vi "DMM.vi"(11 "Queue Ref In":T1={"UI"=refnum, "Message"=refnum, "Data"=refnum, "Caller"=refnum, "Name"="000 Common", "Data Path"=path "", "Class Path"=path "", "SubPanel"=refnum, "Project Name"="", "MNT"="", "Title"="", "Data Source"=refnum, "Queue List"={}, "VI"=refnum, "UE"=refnum}) -> ()   [LabVIEW 2020]
doc: "Digital Multimeter"
uses:
  <vilib>/Retry/UI Control Suite/Boolean/System Buttons/Connect Button.ctl
  <vilib>/Retry/UI Control Suite/Boolean/System Buttons/Acquire Button.ctl
  <vilib>/Retry/UI Control Suite/Boolean/System Buttons/Upload Button.ctl
  <vilib>/Retry/UI Control Suite/Boolean/System Buttons/Update Button.ctl
  <vilib>/Retry/UI Control Suite/Boolean/System Buttons/Excel Button.ctl
  <vilib>/Retry/MListBox/MListBox.lvclass
  <vilib>/Retry/MListBox/Type Definitions/Autosize Mode.ctl
  <vilib>/Retry/MListBox/MListBox.lvclass/MListBox.ctl
  <userlib>/_OpenG.lib/array/array.llb/Filter 1D Array with Scalar (I32)__ogtk.vi
  <userlib>/_OpenG.lib/array/array.llb/Sort 2D Array (String)__ogtk.vi
  Spire.XLS.dll
  <vilib>/Retry/Spire Excel/Spire_Excel.lvlib
  <instrlib>/Fluke 5XXX Series Multicalibrators/Fluke 5XXX Series Multicalibrators.lvlib
panel:
  in  "待选参数":i32[](listbox)
  in  "Title":string="数字多用表自动化计量软件V1.0"
  in  "打开报告":T2
  in  "复位":T3
  in  "暂停":bool
  in  "测量参数":T4={"电阻"=TRUE, "直流电压"=TRUE, "交流电压"=TRUE, "直流电流"=TRUE, "交流电流"=TRUE}
  in  "样品编号":string
  in  "载入模版":T5
  in  "型号":u16(ring) items=["34401A", "34461A", "Simulation DMM"]
  in  "保存":bool
  in  "测量":T6
  out "Connected?":bool
  in  "连接":T7
  in  "源地址":refnum<visa-resource-name>="GPIB0::4::INSTR"
  in  "数表地址":refnum<visa-resource-name>
  in  "Tab Control":enum32{"直流电压", "直流电流", "交流电压", "交流电流", "电阻"}(tab)
  in  "直流电压_MLb":i32(listbox)
  in  "直流电流_MLb":i32(listbox)
  in  "交流电压_MLb":i32(listbox)
  in  "交流电流_MLb":i32(listbox)
  in  "电阻_MLb":i32(listbox)
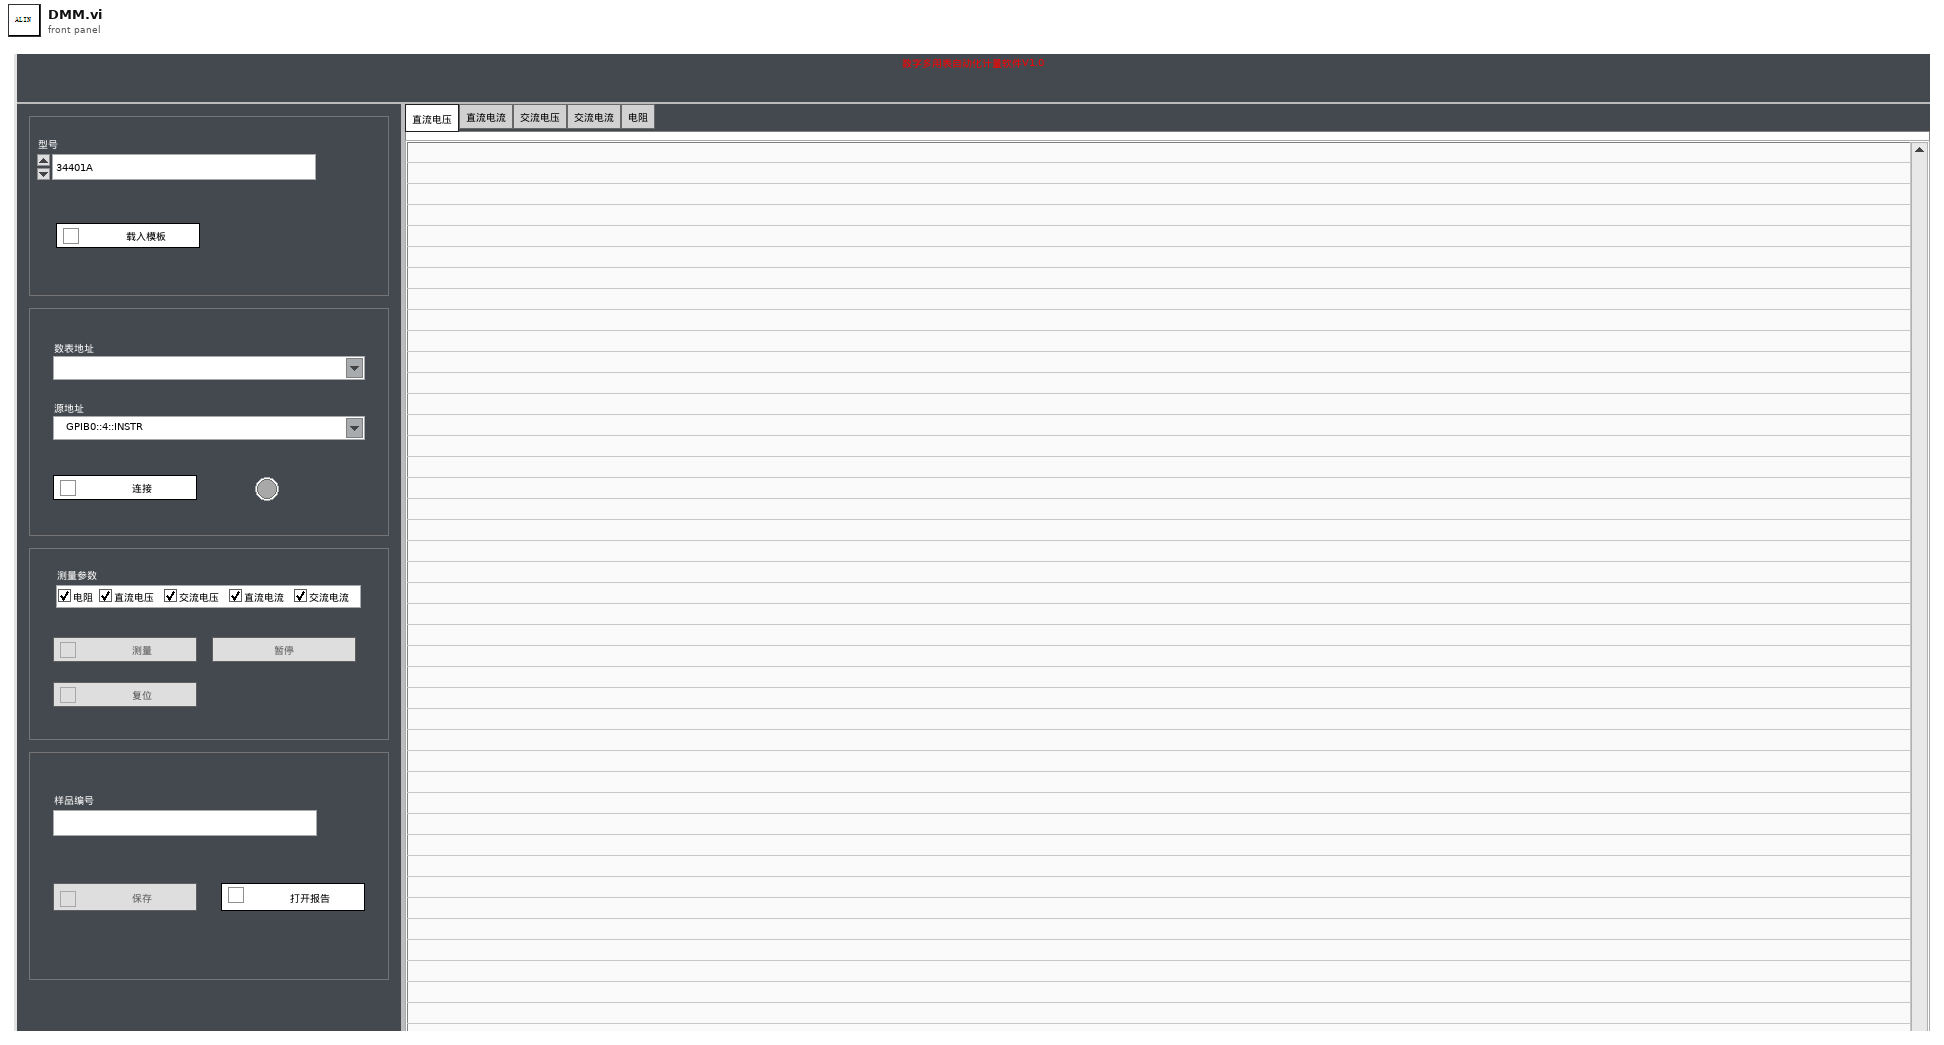
[diagram p1: front panel]
types:
  T1 = typedef "000 Module Data Type.ctl" = cluster{"UI":refnum<queue>, "Message":refnum<queue>, "Data":refnum<queue>, "Caller":refnum<queue>, "Name":string, "Data Path":path, "Class Path":path, "SubPanel":refnum<vi>, "Project Name":string, "MNT":string, "Title":string, "Data Source":refnum<queue>, "Queue List":map{string, refnum<queue>}, "VI":refnum<vi>, "UE":refnum<user-event>}
  T2 = typedef "Excel Button.ctl" = bool
  T3 = typedef "Update Button.ctl" = bool
  T4 = cluster{"电阻":bool, "直流电压":bool, "交流电压":bool, "直流电流":bool, "交流电流":bool}
  T5 = typedef "Upload Button.ctl" = bool
  T6 = typedef "Acquire Button.ctl" = bool
  T7 = typedef "Connect Button.ctl" = bool
  T8 = cluster{"Queue":T1, "Delay":cluster{"Count Time(ms)":u32, "Delay Time(ms)":u32, "Next":string}, "connection ID":refnum<k5>, "Save path":path, "testCount":u32, "数字多用表接口":refnum<class "数字多用表接口.lvclass">, "多功能校准源接口":refnum<class "多功能校准源接口.lvclass">, "workbook":refnum<k24>, "点数范围":string[][], "参数个数":string[], "当前参数":string, "个数索引":i32, "配置数组":string[][], "Measurement":dbl, "MLbs":refnum<class "MListBox.lvclass">[], "测量参数":refnum<vi>, "测量参数s":string[], "参数索引":i32, "接线状态":cluster{"上次接线状态":i32, "当前接线状态":i32}, "MListBox":refnum<class "MListBox.lvclass">, "初始化数据":string[][][], "Message":string, "Delay Time(ms)":u32, "MeaCount":i32, "Restart":bool}
  T9 = enum8{"Enabled", "Disabled", "Disabled and Grayed Out"}
  T10 = enum16{"DC Voltage", "AC Voltage", "Resistance", "DC Current", "AC Current"}
  T11 = typedef "Autosize Mode.ctl" = enum16{"Header", "All Cells"}
  T12 = cluster{"MListBox":refnum<class "MListBox.lvclass">, "Values":string[][]}
  T13 = cluster{"Queue":T1, "MLbs":refnum<class "MListBox.lvclass">[], "MListBox":refnum<class "MListBox.lvclass">}
  T14 = enum32{"invalid app kind", "Development System", "Run Time System", "Student Edition", "Embedded LabVIEW", "Evaluation", "Custom"}
  T15 = typedef "eventvkey.ctl" = enum16{"ASCII", "Enter", "Return", "Shift", "Ctrl", "Alt", "Cmd", "Opt", "Caps", "NumLock", "Clear", "Break", "Up", "Down", "Left", "Right", "Insert", "Delete", "Home", "End", "PageUp", "PageDown", "Escape", "Help", "Pause", "ScrollLock", "F1", "F2", "F3", "F4", "F5", "F6", "F7", "F8", "F9", "F10", "F11", "F12", "F13", "F14", "F15", "F16", "F17", "F18", "F19", "F20", "F21", "F22", "F23", "F24", "Play", "VolumeUp", "VolumeDown", "Mute", "Two Byte Char"}
  T16 = cluster{"Shift":bool, "Ctrl":bool, "Alt":bool, "Cmd":bool, "Opt":bool}
  T17 = typedef "LVPoint32TypeDef.ctl" = cluster{"Horizontal":i32, "Vertical":i32}
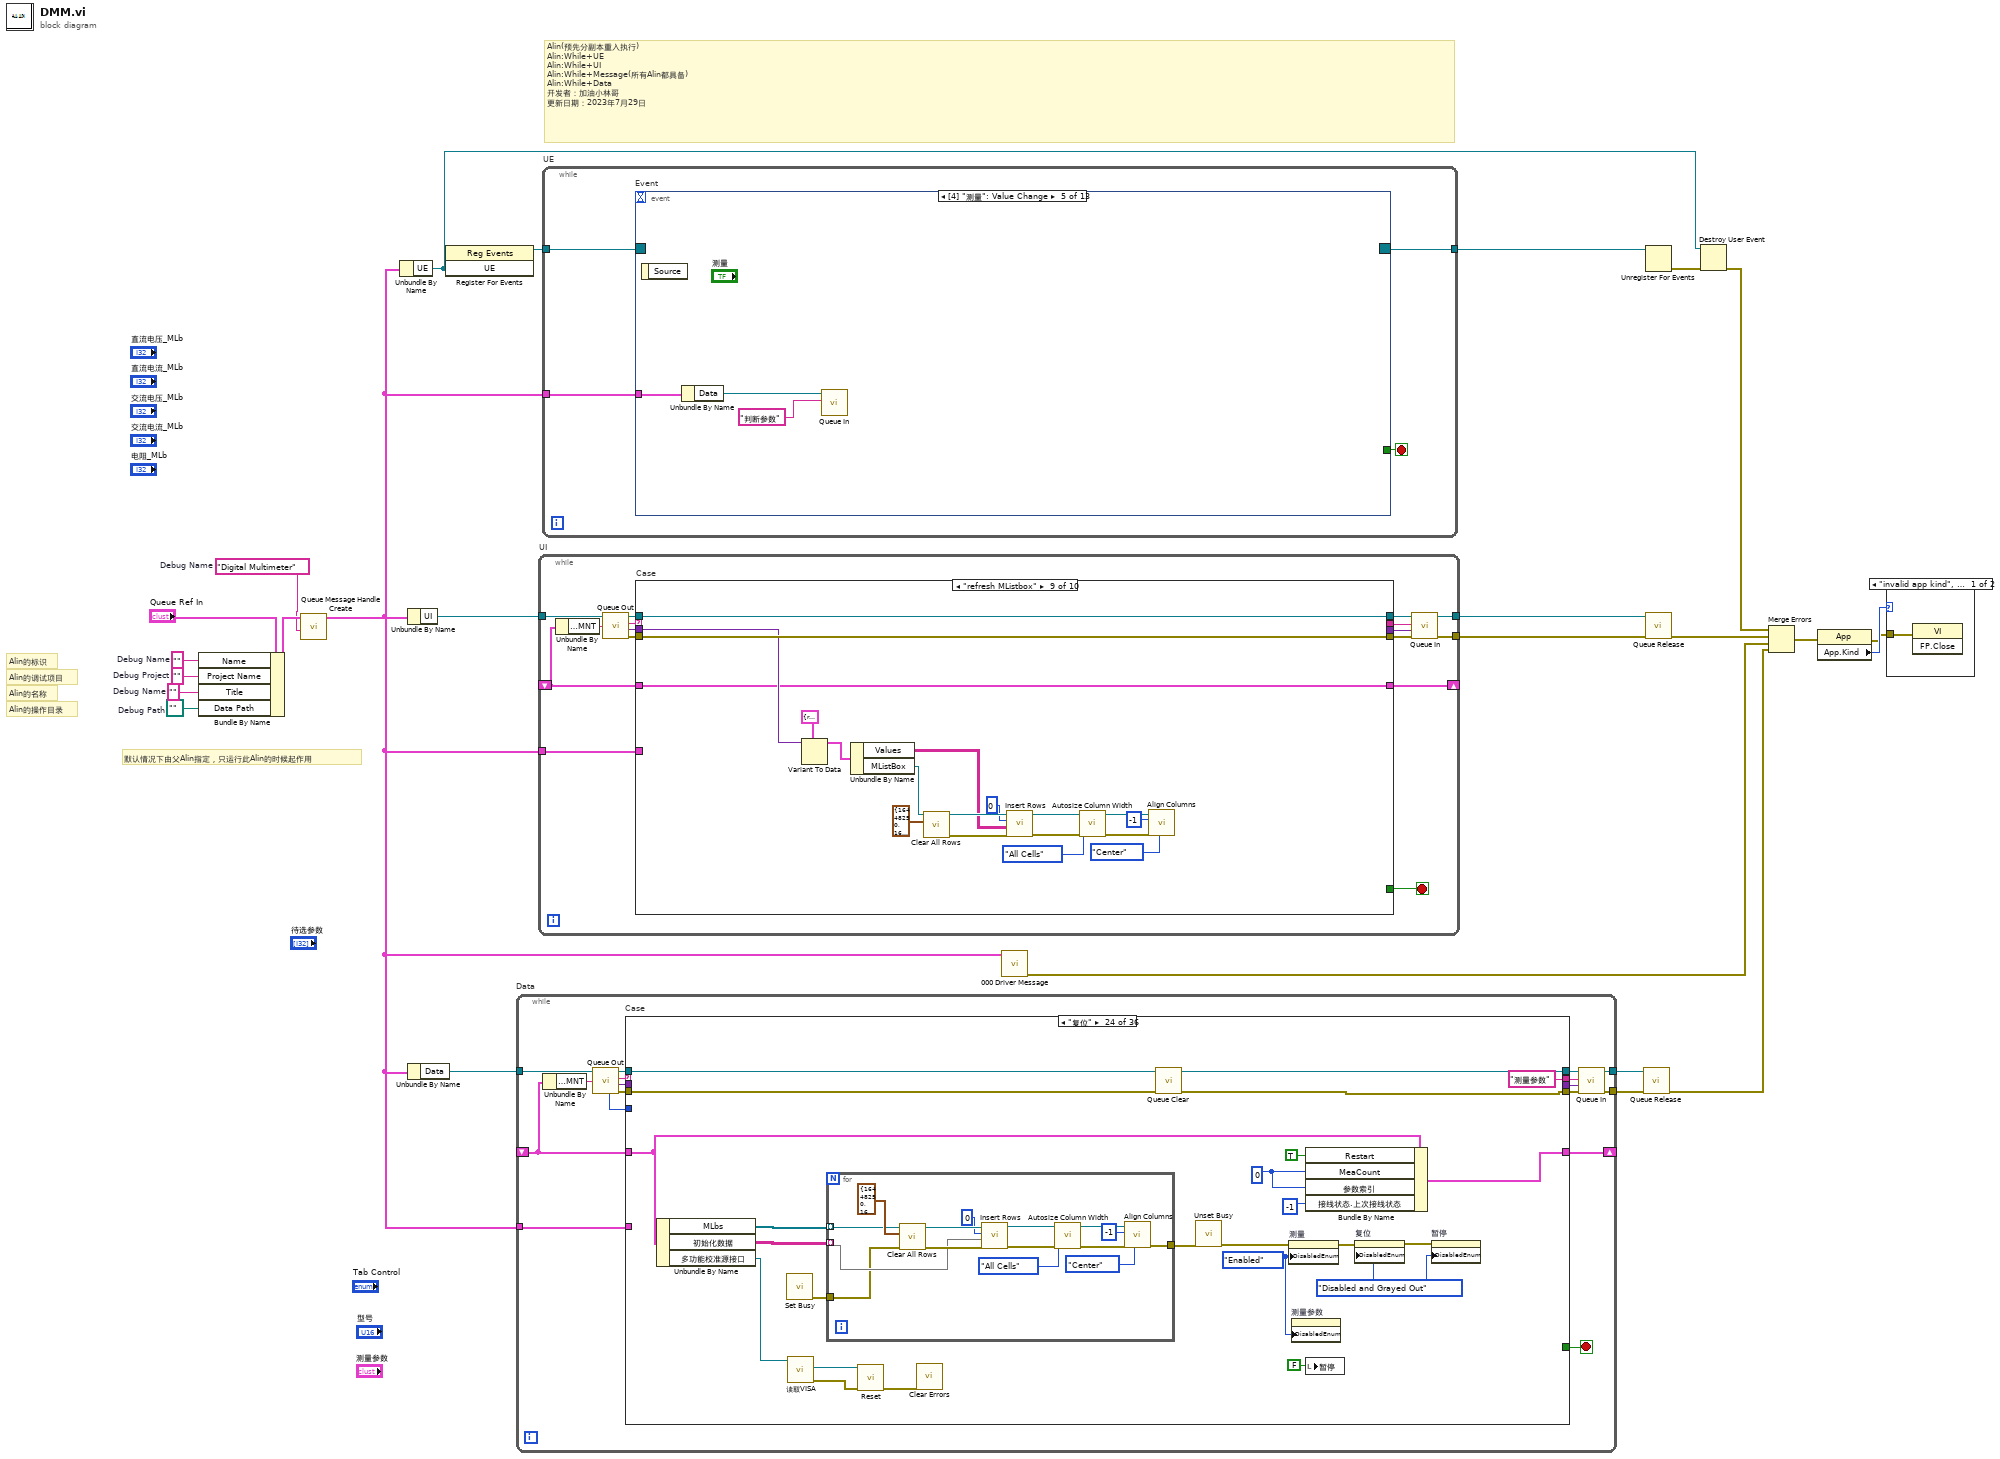
[diagram p0: block diagram]
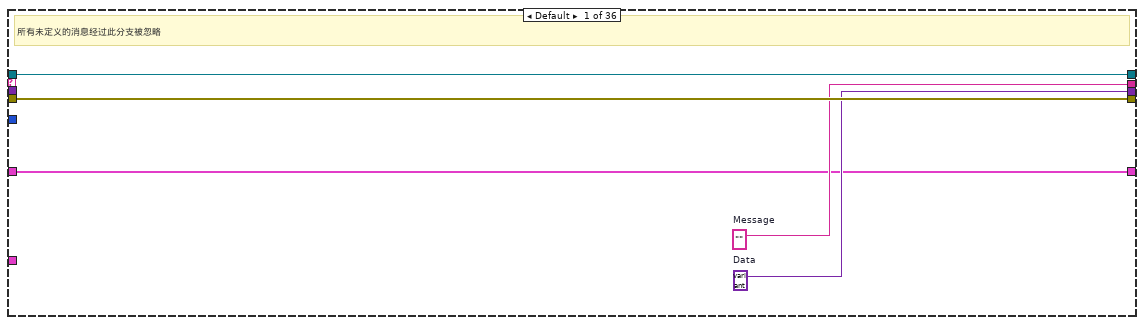
[diagram p3: hidden frame]
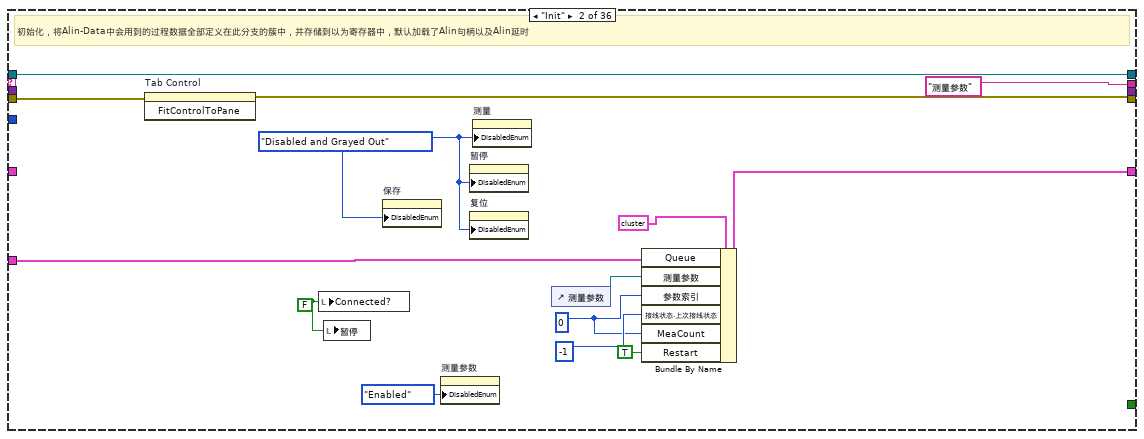
[diagram p4: hidden frame]
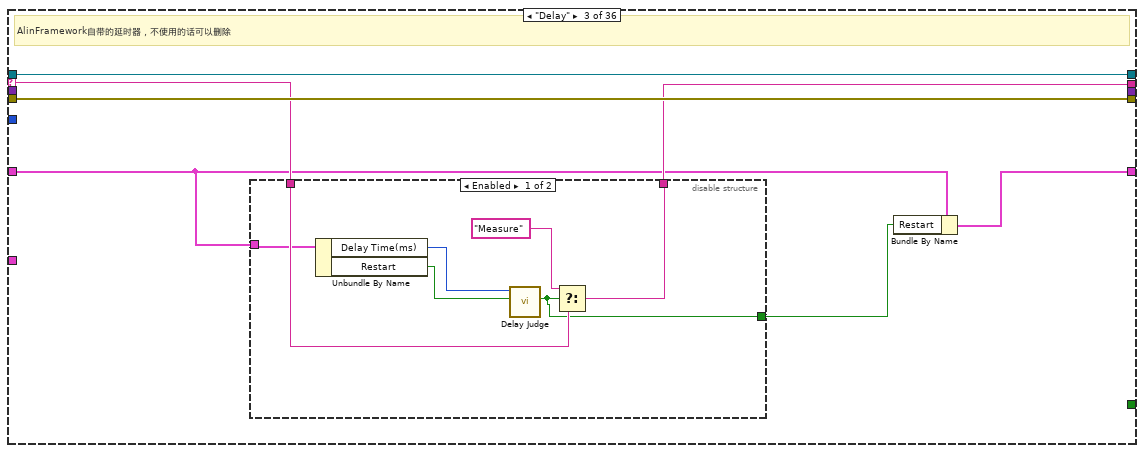
[diagram p5: hidden frame]
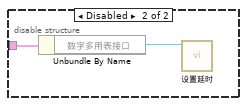
[diagram p6: hidden frame]
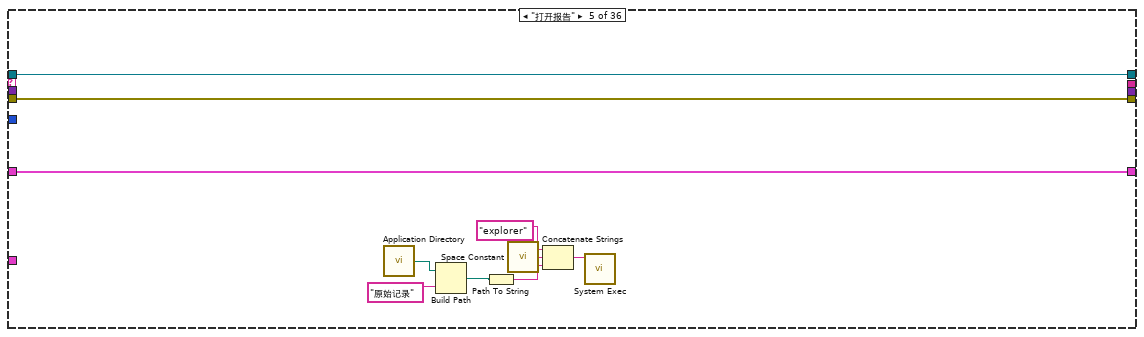
[diagram p8: hidden frame]
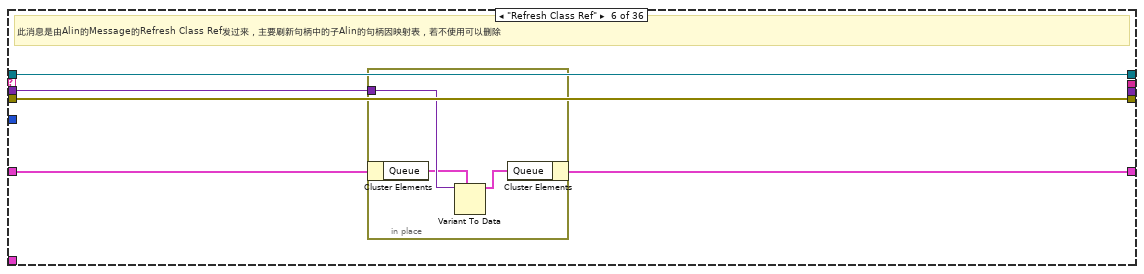
[diagram p9: hidden frame]
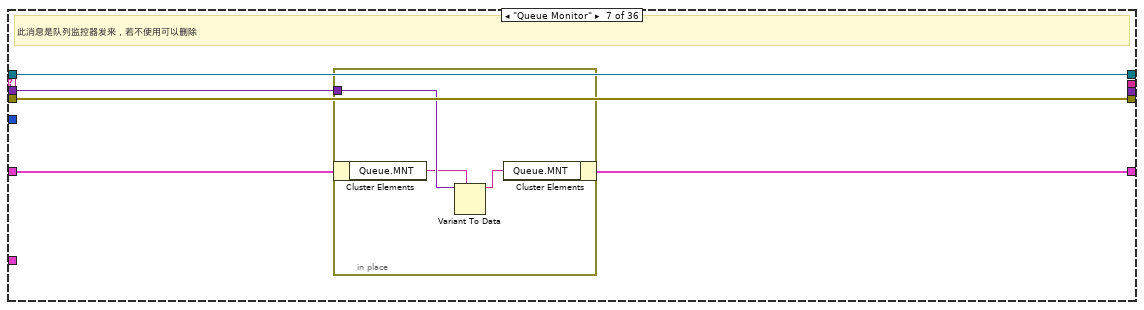
[diagram p10: hidden frame]
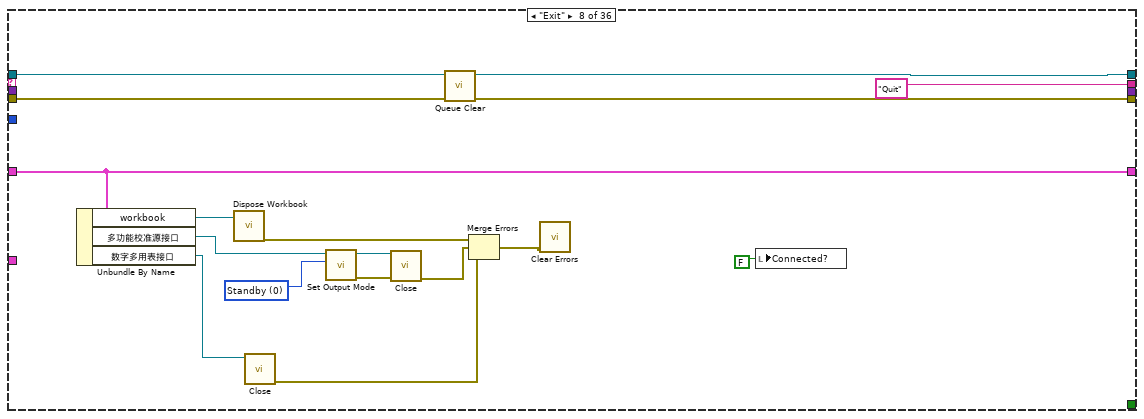
[diagram p11: hidden frame]
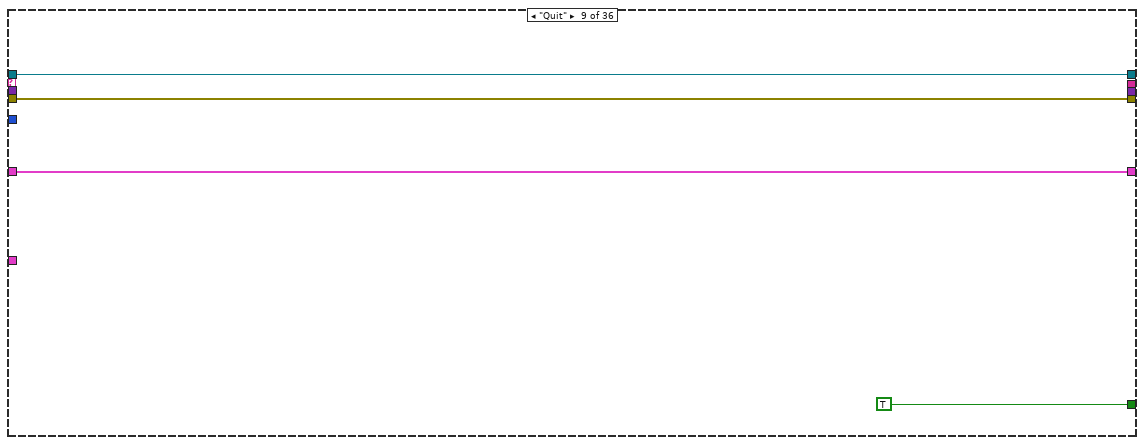
[diagram p12: hidden frame]
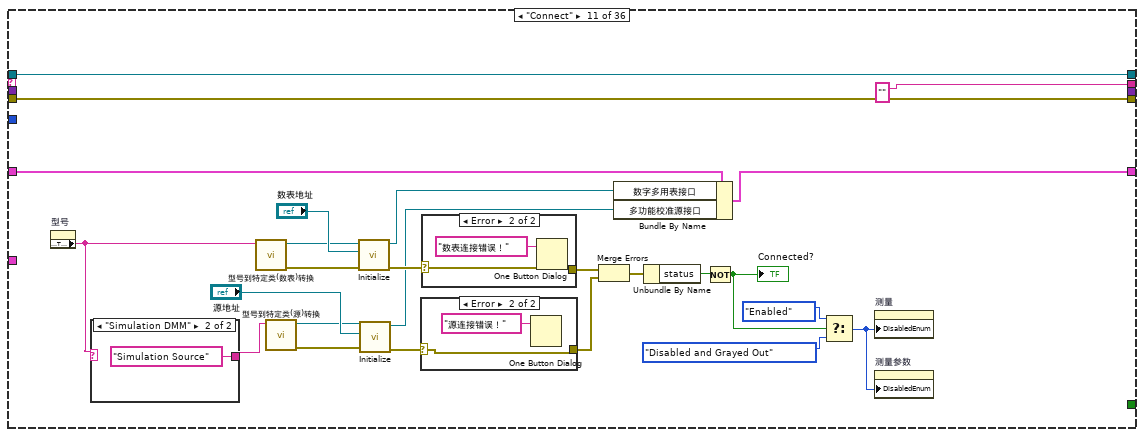
[diagram p14: hidden frame]
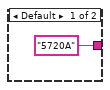
[diagram p15: hidden frame]
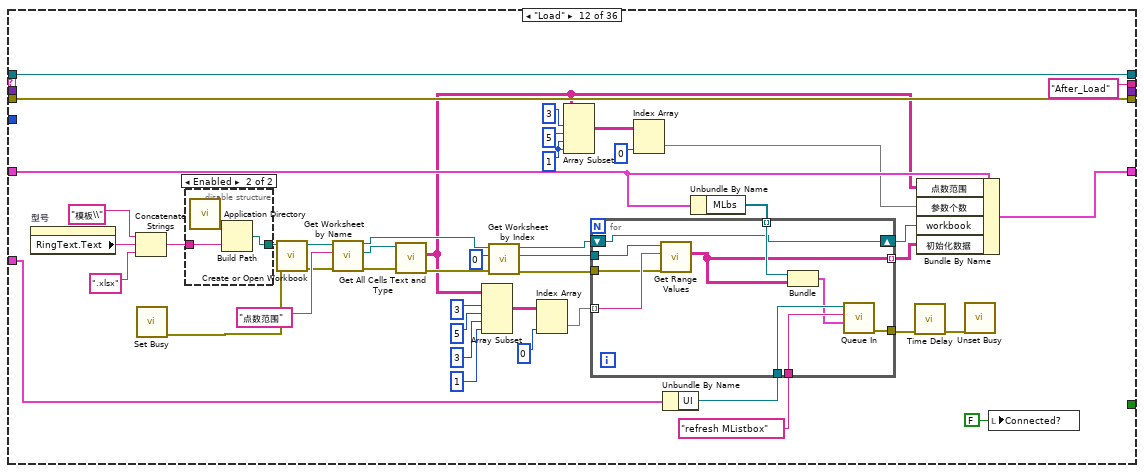
[diagram p18: hidden frame]
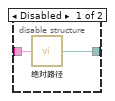
[diagram p19: hidden frame]
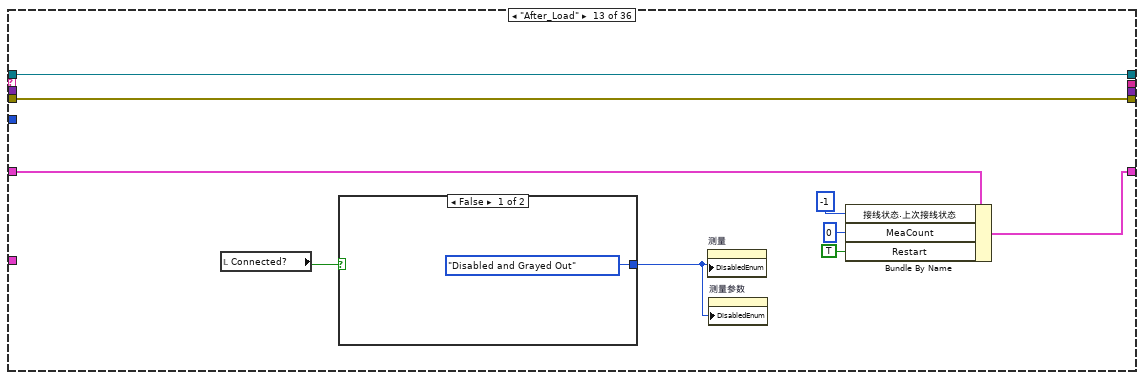
[diagram p20: hidden frame]
diagram:
  w1 = "Digital Multimeter"  # Debug Name
  w5 = ""  # Debug Name
  w6 = ""  # Debug Project
  w7 = path ""  # Debug Path
  w8 = ""  # Debug Name
  # "Alin(预先分副本重入执行)\nAlin:While+UE\nAlin:While+UI\nAlin:While+Message(所有Alin都具备)\nAlin:While+Data\n开发者：加油小林哥\n更新日期：2023年7月29日"
  # "默认情况下由父Alin指定，只运行此Alin的时候起作用"
  # "Alin的标识"
  # "Alin的调试项目"
  # "Alin的名称"
  # "Alin的操作目录"
  n1 = Bundle By Name ("按名称捆绑")(cluster="Queue Ref In", "Name"=w5, "Project Name"=w6, "Title"=w8, "Data Path"=w7) -> (w9:T1)
  n2 = call "Queue Message Handle Create.vi"("Name"=w1, "Queue Ref In"=w9) -> ("Queue Ref Out"=w10:T1)  [unwired: 7 in, 2 out]
  n3 = Unbundle By Name ("按名称解除捆绑")(w10) -> ("UE"=w12:refnum<user-event>)
  n4 = Unbundle By Name ("按名称解除捆绑")(w10) -> ("UI"=w20:refnum<queue>)
  n5 = Unbundle By Name ("按名称解除捆绑")(w10) -> ("Data"=w15:refnum<queue>)
  n6 = register-events ("注册事件")(w12) -> (reference out=w25:refnum<event-registration>)  [unwired: 2 in, 1 out]
  n7 = while "Data" {
    tunnel: w15 -> [w38]
    tunnel: [w35] -> w17
    tunnel: [w34] -> w16
    shift-right: [w30] -> _
    shift-left: _ -> [w27]
    tunnel: w10 -> [w26]
    stop <- w42 stop-if-true
    n8 = Unbundle By Name ("按名称解除捆绑")(w27) -> ("Queue.MNT"=w28:string)
    n9 = call "Queue Out.vi"("Monitor"=w28, "Queue In"=w38) -> ("error out"=w41:errorcluster, "Data"=w39:variant, "Message"=w40:string, "Queue Out"=w37:refnum<queue>, "Queue NUmber"=w29:i32)  [unwired: 5 in]
    n10 = case "Case" shown="\"复位\"" w40 {
      selector: w40 -> [_ _ w65 _ _ _ _ _ _ _ _ _ _ _ _ _ _ _ _ _ _ _ _ _ _ _ _ _ _ _ _ w557 _ _ _ _]
      tunnel: w37 -> [w47 w61 w68 w80 w90 w95 w103 w122 w126 w130 w155 w208 w232 w243 w271 w304 w319 w328 w343 w352 w372 w401 w443 w446 w490 w508 w521 w527 w536 w539 w555 w568 w571 w574 w581 w627]
      tunnel: w41 -> [w46 w58 w67 w79 w89 w94 w102 w120 w127 w129 w154 w207 w231 w242 w270 w303 w318 w327 w342 w351 w371 w400 w442 w447 w486 w507 w520 w526 w535 w538 w554 w567 w570 w573 w580 w626]
      tunnel: [w47 w61 w68 w80 w90 w95 w103 w121 w126 w130 w155 w208 w232 w243 w271 w304 w319 w328 w343 w352 w369 w401 w443 w445 w488 w508 w521 w527 w536 w539 w555 w568 w571 w574 w581 w627] -> w36
      tunnel: [w46 w57 w67 w79 w89 w94 w102 w119 w127 w129 w154 w207 w231 w242 w270 w303 w318 w327 w342 w351 w370 w400 w442 w444 w485 w507 w520 w526 w535 w538 w554 w567 w570 w573 w580 w626] -> w33
      tunnel: [w45 "测量参数" ("CMD") w66 _ _ _ _ "Quit" _ _ "" ("CMD") "After_Load" ("CMD") _ _ w258 "换线排序" ("CMD") "判断个数" ("CMD") w322 "选tab" ("CMD") "表配置" ("CMD") _ "After_Save" ("CMD") _ "测量参数" ("CMD") w487 _ "Operate" ("CMD") "Delay" ("CMD") "判断个数" ("CMD") _ "源配置" ("CMD") w556 _ _ _ "Standby" ("CMD")] -> w32
      tunnel: [_ _ _ _ _ _ _ _ TRUE _ _ _ _ _ _ _ _ _ _ _ _ _ _ _ _ _ _ _ _ _ _ _ _ _ _ _] -> w42
      tunnel: [w44 _ _ _ _ _ _ _ _ _ _ _ _ _ _ _ _ _ _ _ _ _ _ _ _ _ _ _ _ _ _ _ _ _ _ _] -> w31
      tunnel: w39 -> [_ _ _ _ _ w91 w99 _ _ _ _ _ _ _ _ _ _ _ _ _ _ _ _ _ _ _ _ _ _ _ _ _ _ _ w579 _]
      tunnel: [w43 w60 w62 w78 w88 w92 w100 w118 w124 w128 w138 w193 w227 w236 w267 w292 w311 w321 w330 w349 w368 w399 w441 w460 w484 w506 w509 w525 w529 w537 w543 w563 w569 w572 w576 w582] -> w30
      tunnel: w27 -> [w43 _ w64 w78 w88 w93 w101 w118 w124 w128 w141 w184 w229 w238 w269 w294 w313 w321 w332 w349 w364 w399 w441 w461 w489 w506 w511 w525 w532 w537 w545 w565 w569 w572 w578 w584]
      tunnel: w29 -> [_ _ _ _ _ _ _ _ _ _ _ _ _ _ _ _ _ _ _ _ _ _ _ _ _ _ _ _ _ _ _ _ _ _ _ _]
      tunnel: w26 -> [_ w59 _ _ _ _ _ _ _ _ _ w194 _ _ _ _ _ _ _ _ _ _ _ _ _ _ _ _ _ _ _ _ _ _ _ _]
      frame Default {
        w44 = variant  # Data
        w45 = ""  # Message
        # "所有未定义的消息经过此分支被忽略"
      }
      frame "Init" {
        w53 = FALSE ("Connected?")
        w51 = T9."Disabled and Grayed Out" ("Disabled")
        w50 = 0 ("参数索引")
        # "初始化，将Alin-Data中会用到的过程数据全部定义在此分支的簇中，并存储到以为寄存器中，默认加载了Alin句柄以及Alin延时"
        n11 = invoke on="Tab Control" class="TabCtl (strict)" method="FitControlToPane"(error in=w58) -> (error out=w57:errorcluster)  [unwired: 2 in, 2 out]
        n12 = local write "Connected?"(w53) -> ()
        n13 = local write "暂停"(w53) -> ()
        n14 = property on="保存" class="Bool"("DisabledEnum"=w51) -> ()  [unwired: 2 in, 2 out]
        n15 = property on="测量参数" class="Clust (strict)"("DisabledEnum"=T9."Enabled" ("Disabled")) -> ()  [unwired: 2 in, 2 out]
        n16 = property on="暂停" class="Bool (strict)"("DisabledEnum"=w51) -> ()  [unwired: 2 in, 2 out]
        n17 = property on="复位" class="Bool"("DisabledEnum"=w51) -> ()  [unwired: 2 in, 2 out]
        n18 = property on="测量" class="Bool"("DisabledEnum"=w51) -> ()  [unwired: 2 in, 2 out]
        n19 = control-ref of="测量参数"() -> (w56:refnum<vi>)
        n20 = Bundle By Name(cluster=T8 {"Queue"={"UI"=refnum, "Message"=refnum, "Data"=refnum, "Caller"=refnum, "Name"="000 Common", "Data Path"=path "", "Class Path"=path "", "SubPanel"=refnum, "Project Name"="", "MNT"="", "Title"="", "Data Source"=refnum, "Queue List"={}, "VI"=refnum, "UE"=refnum}, "Delay"={"Count Time(ms)"=250, "Delay Time(ms)"=250, "Next"="Receive Data,Delay"}, "connection ID"=refnum, "Save path"=path "", "testCount"=250, "数字多用表接口"=refnum, "多功能校准源接口"=refnum, "workbook"=refnum, "点数范围"=[], "参数个数"=[], "当前参数"="", "个数索引"=0, "配置数组"=[], "Measurement"=0.0, "MLbs"=[], "测量参数"=refnum, "测量参数s"=[], "参数索引"=0, "接线状态"={"上次接线状态"=-1, "当前接线状态"=-1}, "MListBox"=refnum, "初始化数据"=[], "Message"="", "Delay Time(ms)"=250, "MeaCount"=0, "Restart"=FALSE}, "Queue"=w59, "测量参数"=w56, "参数索引"=w50, "接线状态.上次接线状态"=-1 ("参数索引"), "MeaCount"=w50, "Restart"=TRUE) -> (w60:T8)
      }
      frame "Delay" {
        # "AlinFramework自带的延时器，不使用的话可以删除"
        n21 = disable-structure shown="Enabled" {
          disable-tunnel: [w75 _] -> w66
          disable-tunnel: w65 -> [w74 _]
          disable-tunnel: w64 -> [w72 w77]
          disable-tunnel: [w70 _] -> w63
          frame Enabled {
            n22 = Unbundle By Name(w72) -> ("Delay Time(ms)"=w71:u32, "Restart"=w69:bool)
            n23 = call "Delay Judge.vi"("Restart"=w69, "Count Time(ms)"=w71) -> ("Time Out?"=w70:bool)  [unwired: 5 in, 4 out]
            n24 = Select(t="Measure", s=w70, f=w74) -> (s? t:f=w75:string)
          }
          frame Disabled {
            n25 = Unbundle By Name(w77) -> ("数字多用表接口"=w76:refnum<class "数字多用表接口.lvclass">)
            n26 = call-dynamic "设置延时.vi"("数字多用表接口 输入"=w76) -> ()  [unwired: 9 in, 2 out]
          }
        }
        n27 = Bundle By Name(cluster=w64, "Restart"=w63) -> (w62:T8)
      }
      frame "====System====" {
      }
      frame "打开报告" {
        n28 = call <vilib>:"Application Directory.vi"() -> ("Application Directory"=w84:path)
        n29 = Build Path(base path=w84, name or relative path="原始记录") -> (appended path=w81:path)
        n30 = Path To String(path=w81) -> (string=w86:string)
        n31 = call <vilib>:"Space Constant.vi"() -> ("String"=w87:string)
        n32 = Concatenate Strings("explorer", w87, w86) -> (w85:string)
        n33 = call <vilib>:"System Exec.vi"("command line"=w85) -> ()  [unwired: 7 in, 4 out]
      }
      frame "Refresh Class Ref" {
        # "此消息是由Alin的Message的Refresh Class Ref发过来，主要刷新句柄中的子Alin的句柄因映射表，若不使用可以删除"
        n34 = in-place {
          in-place-border: w91 -> [w98]
          n35 = in-place-cluster #1(w93) -> ("Queue"=w97:T1)
          n36 = Variant To Data(type=w97, Variant=w98) -> (data=w96:T1)  [unwired: 1 in, 1 out]
          n37 = in-place-cluster #1("Queue"=w96) -> (w92:T8)
        }
      }
      frame "Queue Monitor" {
        # "此消息是队列监控器发来，若不使用可以删除"
        n38 = in-place {
          in-place-border: w99 -> [w106]
          n39 = in-place-cluster #2(w101) -> ("Queue.MNT"=w105:string)
          n40 = Variant To Data(type=w105, Variant=w106) -> (data=w104:string)  [unwired: 1 in, 1 out]
          n41 = in-place-cluster #2("Queue.MNT"=w104) -> (w100:T8)
        }
      }
      frame "Exit" {
        w116 = u32 0 items=["Standby", "Operate"] ("Output Mode")
        n42 = Unbundle By Name(w118) -> ("workbook"=w117:refnum<k24>, "多功能校准源接口"=w115:refnum<class "多功能校准源接口.lvclass">, "数字多用表接口"=w112:refnum<class "数字多用表接口.lvclass">)
        n43 = call <vilib>:"Dispose Workbook.vi"("workbook in"=w117) -> ("error out"=w110:errorcluster)  [unwired: 10 in]
        n44 = call-dynamic "Close.vi"("数字多用表接口 输入"=w112) -> ("error out"=w108:errorcluster)  [unwired: 9 in, 1 out]
        n45 = call-dynamic "Set Output Mode.vi"("Output Mode"=w116, "多功能校准源接口 输入"=w115) -> ("error out"=w113:errorcluster, "多功能校准源接口 输出"=w114:refnum<class "多功能校准源接口.lvclass">)  [unwired: 8 in]
        n46 = call-dynamic "Close.vi"("error in (no error)"=w113, "多功能校准源接口 输入"=w114) -> ("error out"=w109:errorcluster)  [unwired: 8 in, 1 out]
        n47 = call "Queue Clear.vi"("error in (no error)"=w120, "Queue In"=w122) -> ("error out"=w119:errorcluster, "Queue Out"=w121:refnum<queue>)  [unwired: 8 in]
        n48 = Merge Errors(w110, w109, w108) -> (w111:errorcluster)
        n49 = call <vilib>:"Clear Errors.vi"("error in (no error)"=w111) -> ()  [unwired: 5 in, 2 out]
        n50 = local write "Connected?"(FALSE ("Connected?")) -> ()
      }
      frame "Quit" {
      }
      frame "====User====" {
      }
      frame "Connect" {
        n51 = property on="型号" class="Ring (strict)"() -> ("RingText.Text"=w132:string)  [unwired: 2 in, 2 out]
        n52 = case shown="\"Simulation DMM\"" w132 {
          tunnel: ["5720A" ("型号") "Simulation Source" ("型号")] -> w131
          frame Default {
          }
          frame "Simulation DMM" {
          }
        }
        n53 = call "型号到特定类(数表)转换.vi"("型号"=w132) -> ("错误输出"=w148:errorcluster, "DMM"=w149:refnum<class "数字多用表接口.lvclass">)  [unwired: 9 in]
        n54 = call "型号到特定类(源)转换.vi"("型号"=w131) -> ("错误输出"=w151:errorcluster, "MC"=w152:refnum<class "多功能校准源接口.lvclass">)  [unwired: 9 in]
        n55 = call-dynamic "Initialize.vi"("error in (no error)"=w148, "VISA资源名称"="数表地址", "数字多用表接口 输入"=w149) -> ("error out"=w147:errorcluster, "数字多用表接口 输出"=w140:refnum<class "数字多用表接口.lvclass">)  [unwired: 7 in]
        n56 = call-dynamic "Initialize.vi"("error in (no error)"=w151, "多功能源VISA"="源地址", "多功能校准源接口 输入"=w152) -> ("error out"=w146:errorcluster, "多功能校准源接口 输出"=w139:refnum<class "多功能校准源接口.lvclass">)  [unwired: 7 in]
        n57 = case shown="Error" w146 {
          selector: w146 -> [w158 w159]
          tunnel: [w158 w159] -> w144
          frame No Error {
          }
          frame Error {
            n58 = One Button Dialog(message="源连接错误！" ("消息")) -> ()  [unwired: 1 in, 1 out]
          }
        }
        n59 = case shown="Error" w147 {
          selector: w147 -> [w161 w162]
          tunnel: [w161 w162] -> w145
          frame No Error {
          }
          frame Error {
            n60 = One Button Dialog(message="数表连接错误！" ("消息")) -> ()  [unwired: 1 in, 1 out]
          }
        }
        n61 = Merge Errors(w145, w144) -> (w143:errorcluster)
        n62 = Bundle By Name(cluster=w141, "数字多用表接口"=w140, "多功能校准源接口"=w139) -> (w138:T8)
        n63 = Unbundle By Name(w143) -> ("status"=w142:bool)
        n64 = Not(x=w142) -> (.not. x?=w135:bool)
        "Connected?" <- w135
        n65 = Select(t=T9."Enabled" ("Disabled"), s=w135, f=T9."Disabled and Grayed Out" ("Disabled")) -> (s? t:f=w133:T9)
        n66 = property on="测量" class="Bool"("DisabledEnum"=w133) -> ()  [unwired: 2 in, 2 out]
        n67 = property on="测量参数" class="Clust (strict)"("DisabledEnum"=w133) -> ()  [unwired: 2 in, 2 out]
      }
      frame "Load" {
        w174 = 1 ("index")
        n68 = property on="型号" class="Ring (strict)"() -> ("RingText.Text"=w195:string)  [unwired: 2 in, 2 out]
        n69 = Concatenate Strings("模板\\" ("string"), w195, ".xlsx" ("string")) -> (w197:string)
        n70 = call <vilib>:"Set Busy.vi"() -> ("error out"=w169:errorcluster)  [unwired: 10 in, 1 out]
        n71 = disable-structure shown="Enabled" {
          disable-tunnel: w197 -> [w210 w212]
          disable-tunnel: [w209 w211] -> w192
          frame Disabled {
            n72 = call "绝对路径.vi"("相对路径"=w210) -> ("绝对路径"=w209:path)
          }
          frame Enabled {
            n73 = call <vilib>:"Application Directory.vi"() -> ("Application Directory"=w213:path)
            n74 = Build Path(base path=w213, name or relative path=w212) -> (appended path=w211:path)
          }
        }
        n75 = call <vilib>:"Create or Open Workbook.vi"("error in (no error)"=w169, "file path"=w192) -> ("error out"=w191:errorcluster, "workbook out"=w199:refnum<k24>)  [unwired: 8 in]
        n76 = call <vilib>:"Get Worksheet by Name.vi"("error in (no error)"=w191, "name"="点数范围", "workbook in"=w199) -> ("error out"=w201:errorcluster, "worksheet"=w202:refnum<k24>, "workbook out"=w182:refnum<k24>)  [unwired: 6 in]
        n77 = call <vilib>:"Get All Cells Text and Type.vi"("error in (no error)"=w201, "worksheet in"=w202) -> ("error out"=w181:errorcluster, "texts"=w170:string[][])  [unwired: 6 in, 2 out]
        n78 = Array Subset(array=w170, index (row)=3 ("index"), length (row)=5 ("index"), index (col)=3 ("index"), length (col)=1 ("index")) -> (w190:string[][])
        n79 = call <vilib>:"Get Worksheet by Index.vi"("error in (no error)"=w181, "index"=0, "workbook in"=w182) -> ("error out"=w179:errorcluster, "worksheet"=w177:refnum<k24>, "workbook out"=w178:refnum<k24>)  [unwired: 6 in]
        n80 = Index Array(array=w190, index (col)=0 ("disabled index (col)")) -> (element=w188:string[])  [unwired: 1 in]
        n81 = Array Subset(array=w170, index (row)=3 ("index"), length (row)=5 ("index"), index (col)=w174, length (col)=w174) -> (w172:string[][])
        n82 = Index Array(array=w172, index (col)=0 ("disabled index (col)")) -> (element=w171:string[])  [unwired: 1 in]
        n83 = Unbundle By Name(w194) -> ("UI"=w185:refnum<queue>)
        n84 = Unbundle By Name(w184) -> ("MLbs"=w183:refnum<class "MListBox.lvclass">[])
        n85 = for {
          tunnel: w188 -> [w223] mode=indexing
          tunnel: w179 -> [w216]
          shift-right: [w217] -> w187
          shift-left: w178 -> [w217]
          tunnel: "refresh MListbox" ("Message") -> [w222]
          tunnel: w185 -> [w221]
          tunnel: w183 -> [w220] mode=indexing
          tunnel: w177 -> [w218]
          tunnel: [w215] -> w168
          tunnel: [w214] -> w166 mode=indexing
          n86 = call "Get Range Values.vi"("error in (no error)"=w216, "Cell:Cell"=w223, "worksheet in"=w218) -> ("Values"=w214:string[][])  [unwired: 6 in, 2 out]
          n87 = Bundle("MListBox"=w220, "Values"=w214) -> (w219:T12)  [unwired: 1 in]
          n88 = call "Queue In.vi"("Data"=w219, "Message"=w222, "Queue In"=w221) -> ("error out"=w215:errorcluster)  [unwired: 7 in, 1 out]
        }
        n89 = call "Time Delay"("error in (no error)"=w168) -> ("error out"=w167:errorcluster)  [unwired: 10 in]
        n90 = Bundle By Name(cluster=w184, "点数范围"=w170, "参数个数"=w171, "workbook"=w187, "初始化数据"=w166) -> (w193:T8)
        n91 = call <vilib>:"Unset Busy.vi"("error in (no error)"=w167) -> ()  [unwired: 10 in, 1 out]
        n92 = local write "Connected?"(FALSE ("Connected?")) -> ()
      }
      frame "After_Load" {
        n93 = local read "Connected?"() -> (w230:bool)
        n94 = case shown="False" w230 {
          tunnel: [T9."Disabled and Grayed Out" ("Disabled") T9."Enabled" ("Disabled")] -> w226
          frame False {
          }
          frame True {
          }
        }
        n95 = property on="测量" class="Bool"("DisabledEnum"=w226) -> ()  [unwired: 2 in, 2 out]
        n96 = property on="测量参数" class="Clust (strict)"("DisabledEnum"=w226) -> ()  [unwired: 2 in, 2 out]
        n97 = Bundle By Name(cluster=w229, "接线状态.上次接线状态"=-1, "MeaCount"=0, "Restart"=TRUE) -> (w227:T8)
      }
      frame "测量参数" {
        n98 = Unbundle By Name(w238) -> ("测量参数"=w239:refnum<vi>)
        n99 = property class="Clust (strict)"(reference=w239) -> ("Controls[]"=w240:refnum<vi>[])  [unwired: 1 in, 2 out]
        n100 = for {
          shift-right: [w245] -> w237
          shift-left: string[] [] ("数组") -> [w246]
          tunnel: w240 -> [w244] mode=indexing
          n101 = property class="Ctl"(reference=w244) -> ("Label.Text"=w247:string, "Value"=w250:variant)  [unwired: 1 in, 2 out]
          n102 = Variant To Data(type=TRUE, Variant=w250) -> (data=w248:bool)  [unwired: 1 in, 1 out]
          n103 = case shown="True" w248 {
            tunnel: w247 -> [_ w253]
            tunnel: w246 -> [w251 w254]
            tunnel: [w251 w252] -> w245
            frame False {
            }
            frame True {
              n104 = Insert Into Array(array=w254, new element=w253) -> (w252:string[])  [unwired: 1 in]
            }
          }
        }
        n105 = Bundle By Name(cluster=w238, "测量参数s"=w237, "参数索引"=0) -> (w236:T8)
      }
      frame "判断参数" {
        n106 = Unbundle By Name(w269) -> ("测量参数s"=w263:string[], "参数索引"=w260:i32, "数字多用表接口"=w266:refnum<class "数字多用表接口.lvclass">, "MLbs"=w257:refnum<class "MListBox.lvclass">[])
        n107 = Index Array(array=w263, index=w260) -> (element=w256:string)
        n108 = for {
          tunnel: w257 -> [w278] mode=indexing
          tunnel: w256 -> [w275]
          tunnel: [w277] -> w255
          stop <- w273 stop-if-true
          n109 = call <vilib>:"Get MListbox Ref.vi"("Multicolumn ListBox in"=w278) -> ("error out"=w272:errorcluster, "MListbox Ref"=w279:refnum<vi>, "Multicolumn ListBox out"=w277:refnum<class "MListBox.lvclass">)  [unwired: 8 in]
          n110 = property class="MCListbox (strict)"(reference=w279, error in=w272) -> ("Label.Text"=w276:string)  [unwired: 2 out]
          n111 = Search and Replace String(input string=w276, search string=w275) -> (number of replacements=w274:i32)  [unwired: 6 in, 3 out]
          n112 = Not Equal To 0?(x=w274) -> (x != 0?=w273:bool)
        }
        n113 = Array Size(array=w263) -> (size(s)=w261:i32)
        n114 = case shown="\"电阻\", Default" w256 {
          tunnel: [T10."Resistance" ("测量参数") T10."DC Voltage" ("测量参数") T10."AC Voltage" ("测量参数") T10."DC Current" ("测量参数") T10."AC Current" ("测量参数")] -> w265
          frame "电阻", Default {
          }
          frame "直流电压" {
          }
          frame "交流电压" {
          }
          frame "直流电流" {
          }
          frame "交流电流" {
          }
        }
        n115 = Equal?(x=w261, y=w260) -> (x = y?=w259:bool)
        n116 = Increment(x=w260) -> (x+1=w262:i32)
        n117 = call "写入测量参数.vi"("测量参数"=w265, "数字多用表接口输入"=w266) -> ("数字多用表接口输出"=w264:refnum<class "数字多用表接口.lvclass">)  [unwired: 8 in, 1 out]
        n118 = Bundle By Name(cluster=w269, "当前参数"=w256, "参数索引"=w262, "个数索引"=0, "数字多用表接口"=w264, "MListBox"=w255) -> (w267:T8)
        n119 = case shown="False" w259 {
          tunnel: ["读配置" "End Test"] -> w258
          frame False {
          }
          frame True {
          }
        }
      }
      frame "读配置" {
        w287 = T9."Disabled and Grayed Out" ("Disabled")
        n120 = Unbundle By Name(w294) -> ("workbook"=w300:refnum<k24>, "当前参数"=w290:string, "参数个数"=w297:string[])
        n121 = case shown="\"电阻\", Default" w290 {
          tunnel: [4 0 2 1 3] -> w289
          frame "电阻", Default {
          }
          frame "直流电压" {
          }
          frame "交流电压" {
          }
          frame "直流电流" {
          }
          frame "交流电流" {
          }
        }
        n122 = Index Array(array=w297, index=w289) -> (element=w295:string)
        n123 = call <vilib>:"Get Worksheet by Name.vi"("name"=w290, "workbook in"=w300) -> ("error out"=w301:errorcluster, "worksheet"=w302:refnum<k24>)  [unwired: 7 in, 1 out]
        n124 = Decimal String To Number(string=w295) -> (number=w293:i32)  [unwired: 2 in, 1 out]
        n125 = call <vilib>:"Get All Cells Text and Type.vi"("error in (no error)"=w301, "worksheet in"=w302) -> ("texts"=w298:string[][])  [unwired: 6 in, 3 out]
        n126 = Array Subset(array=w298, index (row)=1 ("index"), length (row)=w293) -> (w291:string[][])  [unwired: 2 in]
        n127 = Bundle By Name(cluster=w294, "testCount"=w293, "配置数组"=w291) -> (w292:T8)
        n128 = property on="暂停" class="Bool (strict)"("DisabledEnum"=T9."Enabled" ("Disabled")) -> ()  [unwired: 2 in, 2 out]
        n129 = property on="测量" class="Bool"("DisabledEnum"=w287) -> ()  [unwired: 2 in, 2 out]
        n130 = property on="测量参数" class="Clust (strict)"("DisabledEnum"=w287) -> ()  [unwired: 2 in, 2 out]
        n131 = property on="保存" class="Bool"("DisabledEnum"=w287) -> ()  [unwired: 2 in, 2 out]
      }
      frame "换线排序" {
        n132 = Unbundle By Name(w313) -> ("配置数组"=w310:string[][])
        n133 = call-poly <userlib>:"Sort Array__ogtk.vi"("Column/Row to Sort By"=u32 7, "Sort By in"=enum16{"row", "column"}."column", "Order"=enum16{"ascending", "descending"}."ascending", "Array in"=w310) -> ("Sorted Array out"=w312:string[][])  [unwired: 4 in, 3 out]
        n134 = Bundle By Name(cluster=w313, "配置数组"=w312) -> (w311:T8)
      }
      frame "判断个数" {
        n135 = Unbundle By Name(w321) -> ("testCount"=w326:u32, "个数索引"=w325:i32)
        n136 = Equal?(x=w326, y=w325) -> (x = y?=w320:bool)
        n137 = Select(t="判断参数", s=w320, f="换线提示") -> (s? t:f=w322:string)
      }
      frame "换线提示" {
        n138 = Unbundle By Name(w332) -> ("数字多用表接口"=w341:refnum<class "数字多用表接口.lvclass">, "接线状态.上次接线状态"=w334:i32, "配置数组"=w339:string[][], "个数索引"=w335:i32)
        n139 = Index Array(array=w339, index (col)=7 ("disabled index (col)")) -> (element=w337:string[])  [unwired: 1 in]
        n140 = Decimal String To Number(string=w337) -> (number=w336:i32[])  [unwired: 2 in, 1 out]
        n141 = Index Array(array=w336, index=w335) -> (element=w331:i32)
        n142 = property on="型号" class="Ring (strict)"() -> ("RingText.Text"=w329:string)  [unwired: 2 in, 2 out]
        n143 = Not Equal?(x=w334, y=w331) -> (x != y?=w333:bool)
        n144 = case shown="True" w333 {
          tunnel: w341 -> [_ w346]
          tunnel: w331 -> [_ w345]
          tunnel: w329 -> [_ w344]
          frame False {
          }
          frame True {
            n145 = call-dynamic "表换线提示.vi"("型号"=w344, "接线状态"=w345, "数字多用表接口 输入"=w346) -> ()  [unwired: 7 in, 2 out]
          }
        }
        n146 = Bundle By Name(cluster=w332, "接线状态.上次接线状态"=w331) -> (w330:T8)
      }
      frame "选tab" {
        n147 = Unbundle By Name(w349) -> ("当前参数"=w348:string)
        n148 = case shown="\"电阻\", Default" w348 {
          tunnel: [enum32{"直流电压", "直流电流", "交流电压", "交流电流", "电阻"}."电阻" ("Tab Control") enum32{"直流电压", "直流电流", "交流电压", "交流电流", "电阻"}."直流电压" ("Tab Control") enum32{"直流电压", "直流电流", "交流电压", "交流电流", "电阻"}."交流电压" ("Tab Control") enum32{"直流电压", "直流电流", "交流电压", "交流电流", "电阻"}."直流电流" ("Tab Control") enum32{"直流电压", "直流电流", "交流电压", "交流电流", "电阻"}."交流电流" ("Tab Control")] -> w347
          frame "电阻", Default {
          }
          frame "直流电压" {
          }
          frame "交流电压" {
          }
          frame "直流电流" {
          }
          frame "交流电流" {
          }
        }
        n149 = local write "Tab Control"(w347) -> ()
      }
      frame "End Test" {
        w359 = T9."Enabled" ("Disabled")
        w366 = 0 ("个数索引")
        n150 = Unbundle By Name(w364) -> ("多功能校准源接口"=w363:refnum<class "多功能校准源接口.lvclass">)
        n151 = call "读取VISA.vi"("多功能校准源接口输入"=w363) -> ("error out"=w361:errorcluster, "VISA"=w362:refnum<visa-resource-name>)  [unwired: 8 in, 1 out]
        n152 = call <instrlib>:"Reset.vi"("VISA resource name"=w362, "error in (no error)"=w361) -> ("error out"=w360:errorcluster)  [unwired: 13 out]
        n153 = call <vilib>:"Clear Errors.vi"("error in (no error)"=w360) -> ()  [unwired: 5 in, 2 out]
        n154 = call "Queue Clear.vi"("error in (no error)"=w371, "Queue In"=w372) -> ("error out"=w370:errorcluster, "Queue Out"=w369:refnum<queue>)  [unwired: 8 in]
        n155 = Bundle By Name(cluster=w364, "个数索引"=w366, "参数索引"=w366, "接线状态.上次接线状态"=-1 ("个数索引")) -> (w368:T8)
        n156 = One Button Dialog(message="测量完成。") -> ()  [unwired: 1 in, 1 out]
        n157 = property on="测量" class="Bool"("DisabledEnum"=w359) -> ()  [unwired: 2 in, 2 out]
        n158 = property on="复位" class="Bool"("DisabledEnum"=w359) -> ()  [unwired: 2 in, 2 out]
        n159 = property on="测量参数" class="Clust (strict)"("DisabledEnum"=w359) -> ()  [unwired: 2 in, 2 out]
        n160 = property on="保存" class="Bool"("DisabledEnum"=w359) -> ()  [unwired: 2 in, 2 out]
        n161 = property on="暂停" class="Bool (strict)"("DisabledEnum"=T9."Disabled and Grayed Out" ("Disabled")) -> ()  [unwired: 2 in, 2 out]
      }
      frame "Save" {
        (unwired) 7 ("index")
        n162 = Unbundle By Name(w399) -> ("workbook"=w386:refnum<k24>, "MLbs"=w382:refnum<class "MListBox.lvclass">[], "点数范围"=w398:string[][])
        n163 = Array Subset(array=w398, index (row)=3 ("index"), index (col)=8 ("index"), length (col)=6 ("index")) -> (w394:string[][])  [unwired: 1 in]
        n164 = Format Date/Time String(time format string (%c)="%Y-%m-%d %H-%M-%S" ("时间格式字符串(%c)")) -> (date/time string=w392:string)  [unwired: 2 in]
        n165 = call <vilib>:"Get Worksheet by Index.vi"("index"=0, "workbook in"=w386) -> ("error out"=w385:errorcluster, "worksheet"=w384:refnum<k24>, "workbook out"=w381:refnum<k24>)  [unwired: 7 in]
        n166 = for {
          tunnel: w394 -> [w433] mode=indexing
          tunnel: [w416] -> w379
          tunnel: w385 -> [w411]
          tunnel: w384 -> [w412]
          tunnel: w382 -> [w420]
          n167 = Index Array(array=w433) -> (element #1=w421:string, element #2=w432:string, element #3=w426:string, element #4=w413:string, element #5=w410:string, element #6=w409:string)  [unwired: 6 in]
          n168 = case shown="\"交流电压\"" w421 {
            tunnel: [0 1 2 3 4] -> w419
            frame "直流电压", Default {
            }
            frame "直流电流" {
            }
            frame "交流电压" {
            }
            frame "交流电流" {
            }
            frame "电阻" {
            }
          }
          n169 = call <vilib>:"Delimited String to 1D String Array.vi"("delimiter"=",", "delimited string"=w432) -> ("string array"=w430:string[])  [unwired: 9 in]
          n170 = Decimal String To Number(string=w426) -> (number=w425:i32)  [unwired: 2 in, 1 out]
          n171 = Index Array(array=w430) -> (element #1=w429:string, element #2=w428:string)  [unwired: 2 in]
          n172 = Index Array(array=w420, index=w419) -> (element=w418:refnum<class "MListBox.lvclass">)
          n173 = Decimal String To Number(string=w428) -> (number=w423:i32)  [unwired: 2 in, 1 out]
          n174 = Decimal String To Number(string=w429) -> (number=w427:i32)  [unwired: 2 in, 1 out]
          n175 = call <vilib>:"Get All Rows.vi"("Multicolumn ListBox in"=w418) -> ("Array"=w417:string[][])  [unwired: 8 in, 2 out]
          n176 = Array Subset(array=w417, index (row)=w427, length (row)=w425, index (col)=w423, length (col)=1 ("length")) -> (w422:string[][])
          n177 = Fract/Exp String To Number(string=w409) -> (number=w408:dbl)  [unwired: 3 in, 1 out]
          n178 = call <vilib>:"Set Cells Text.vi"("texts"=w422, "start cell name"=w410, "error in (no error)"=w411, "worksheet in"=w412) -> ("error out"=w415:errorcluster, "worksheet out"=w414:refnum<k24>)  [unwired: 6 in]
          n179 = call <vilib>:"Set Rows Height.vi"("error in (no error)"=w415, "row height"=w408, "cell range"=w413, "worksheet in"=w414) -> ("error out"=w416:errorcluster)  [unwired: 6 in, 1 out]
        }
        n180 = property on="型号" class="Ring (strict)"() -> ("RingText.Text"=w390:string)  [unwired: 2 in, 2 out]
        n181 = Format Into String(format string="%s %s %s.xlsx", initial string="原始记录\\" ("string"), w390, "样品编号", w392) -> (resulting string=w374:string)  [unwired: 1 in, 1 out]
        n182 = call <vilib>:"Application Directory.vi"() -> ("Application Directory"=w375:path)
        n183 = for {
          tunnel: string[] ["直流电压", "直流电流", "交流电压", "交流电流", "电阻", "点数范围"] -> [w405] mode=indexing
          shift-right: [w403] -> w378
          shift-left: w379 -> [w404]
          shift-right: [w402] -> w377
          shift-left: w381 -> [w406]
          n184 = call <vilib>:"Delete Worksheet.vi"("error in (no error)"=w404, "name"=w405, "workbook in"=w406) -> ("error out"=w403:errorcluster, "workbook out"=w402:refnum<k24>)  [unwired: 7 in]
        }
        n185 = Build Path(base path=w375, name or relative path=w374) -> (appended path=w373:path)
        n186 = call <vilib>:"Save Workbook.vi"("error in (no error)"=w378, "save as path"=w373, "workbook in"=w377) -> ("error out"=w393:errorcluster)  [unwired: 7 in, 1 out]
        n187 = flat-sequence {
          tunnel: w393 -> [_]
          frame #0 {
            n188 = One Button Dialog(message="保存完成。") -> ()  [unwired: 1 in, 1 out]
          }
        }
      }
      frame "After_Save" {
        w439 = T9."Disabled and Grayed Out" ("Disabled")
        n189 = property on="暂停" class="Bool (strict)"("DisabledEnum"=w439) -> ()  [unwired: 2 in, 2 out]
        n190 = property on="复位" class="Bool"("DisabledEnum"=w439) -> ()  [unwired: 2 in, 2 out]
        n191 = property on="保存" class="Bool"("DisabledEnum"=w439) -> ()  [unwired: 2 in, 2 out]
        n192 = property on="测量" class="Bool"("DisabledEnum"=w439) -> ()  [unwired: 2 in, 2 out]
        n193 = property on="测量参数" class="Clust (strict)"("DisabledEnum"=w439) -> ()  [unwired: 2 in, 2 out]
        n194 = local write "暂停"(FALSE ("暂停")) -> ()
      }
      frame "复位" {
        w457 = T9."Disabled and Grayed Out" ("Disabled")
        w450 = 0 ("参数索引")
        w456 = T9."Enabled" ("Disabled")
        n195 = Unbundle By Name(w461) -> ("MLbs"=w467:refnum<class "MListBox.lvclass">[], "初始化数据"=w466:string[][][], "多功能校准源接口"=w453:refnum<class "多功能校准源接口.lvclass">)
        n196 = call <vilib>:"Set Busy.vi"() -> ("error out"=w465:errorcluster)  [unwired: 10 in, 1 out]
        n197 = call "读取VISA.vi"("多功能校准源接口输入"=w453) -> ("error out"=w454:errorcluster, "VISA"=w455:refnum<visa-resource-name>)  [unwired: 8 in, 1 out]
        n198 = for {
          tunnel: w467 -> [w471] mode=indexing
          tunnel: w466 -> [w470] mode=indexing
          tunnel: w465 -> [w469]
          tunnel: [w468] -> w464
          n199 = call <vilib>:"Clear All Rows.vi"("error in (no error)"=w469, "BackColors"=cluster{"OddRow Color":u32, "EvenRow Color":u32} {"OddRow Color"=16448250, "EvenRow Color"=16448250}, "Multicolumn ListBox in"=w471) -> ("error out"=w481:errorcluster, "Multicolumn ListBox out"=w480:refnum<class "MListBox.lvclass">)  [unwired: 7 in]
          n200 = call <vilib>:"Insert Rows.vi"("error in (no error)"=w481, "Rows"=w470, "Index"=i16 0, "Multicolumn ListBox in"=w480) -> ("error out"=w474:errorcluster, "Multicolumn ListBox out"=w473:refnum<class "MListBox.lvclass">)  [unwired: 5 in, 1 out]
          n201 = call <vilib>:"Autosize Column Width.vi"("error in (no error)"=w474, "Autosize Mode"=Autosize_Mode."All Cells", "Multicolumn ListBox in"=w473) -> ("error out"=w477:errorcluster, "Multicolumn ListBox out"=w476:refnum<class "MListBox.lvclass">)  [unwired: 7 in]
          n202 = call <vilib>:"Align Columns.vi"("Active Cell:Cell Justification"=enum16{"Left", "Center", "Right"}."Center", "error in (no error)"=w477, "Column Index"=i16 -1, "Multicolumn ListBox in"=w476) -> ("error out"=w468:errorcluster)  [unwired: 6 in, 1 out]
        }
        n203 = call <instrlib>:"Reset.vi"("VISA resource name"=w455, "error in (no error)"=w454) -> ("error out"=w452:errorcluster)  [unwired: 13 out]
        n204 = call <vilib>:"Clear Errors.vi"("error in (no error)"=w452) -> ()  [unwired: 5 in, 2 out]
        n205 = call "Queue Clear.vi"("error in (no error)"=w447, "Queue In"=w446) -> ("error out"=w444:errorcluster, "Queue Out"=w445:refnum<queue>)  [unwired: 8 in]
        n206 = call <vilib>:"Unset Busy.vi"("error in (no error)"=w464) -> ("error out"=w463:errorcluster)  [unwired: 10 in]
        n207 = property on="测量" class="Bool"(error in=w463, "DisabledEnum"=w456) -> (error out=w459:errorcluster)  [unwired: 1 in, 1 out]
        n208 = property on="测量参数" class="Clust (strict)"("DisabledEnum"=w456) -> ()  [unwired: 2 in, 2 out]
        n209 = Bundle By Name(cluster=w461, "Restart"=TRUE, "MeaCount"=w450, "参数索引"=w450, "接线状态.上次接线状态"=-1) -> (w460:T8)
        n210 = local write "暂停"(FALSE ("暂停")) -> ()
        n211 = property on="复位" class="Bool"(error in=w459, "DisabledEnum"=w457) -> (error out=w458:errorcluster)  [unwired: 1 in, 1 out]
        n212 = property on="暂停" class="Bool (strict)"(error in=w458, "DisabledEnum"=w457) -> ()  [unwired: 1 in, 2 out]
      }
      frame "暂停" {
        n213 = case shown="True" "暂停" {
          tunnel: w490 -> [w496 w505]
          tunnel: w489 -> [w493 w504]
          tunnel: [w496 w502] -> w488
          tunnel: [w494 "" ("CMD")] -> w487
          tunnel: w486 -> [w495 w500]
          tunnel: [w495 w499] -> w485
          tunnel: [w493 w498] -> w484
          tunnel: [T9."Disabled and Grayed Out" ("Disabled") T9."Enabled" ("Disabled")] -> w483
          frame False {
            n214 = Unbundle By Name(w493) -> ("Message"=w494:string)
          }
          frame True {
            n215 = call "Queue Out.vi"("error in (no error)"=w500, "Queue In"=w505) -> ("error out"=w499:errorcluster, "Message"=w503:string, "Queue Out"=w502:refnum<queue>)  [unwired: 5 in, 2 out]
            n216 = Bundle By Name(cluster=w504, "Message"=w503) -> (w498:T8)
          }
        }
        n217 = property on="复位" class="Bool"("DisabledEnum"=w483) -> ()  [unwired: 2 in, 2 out]
      }
      frame "---------------------源--------------------" {
      }
      frame "源配置" {
        n218 = Unbundle By Name(w511) -> ("当前参数"=w518:string, "多功能校准源接口"=w519:refnum<class "多功能校准源接口.lvclass">, "配置数组"=w517:string[][], "个数索引"=w516:i32)
        n219 = Index Array(array=w517, index (row)=w516) -> (element=w515:string[])  [unwired: 1 in]
        n220 = call "源配置.vi"("Item"=w518, "Arguments"=w515, "多功能校准源接口输入"=w519) -> ("error out"=w514:errorcluster, "多功能校准源接口输出"=w513:refnum<class "多功能校准源接口.lvclass">)  [unwired: 7 in]
        n221 = call-dynamic "Configure.vi"("error in (no error)"=w514, "多功能校准源接口 输入"=w513) -> ("多功能校准源接口 输出"=w510:refnum<class "多功能校准源接口.lvclass">)  [unwired: 8 in, 1 out]
        n222 = Bundle By Name(cluster=w511, "多功能校准源接口"=w510) -> (w509:T8)
      }
      frame "Operate" {
        (unwired) "Delay,Measure" ("CMD")
        w523 = u32 1 items=["Standby", "Operate"] ("Output Mode")
        n223 = Unbundle By Name(w525) -> ("多功能校准源接口"=w524:refnum<class "多功能校准源接口.lvclass">)
        n224 = call-dynamic "Set Output Mode.vi"("Output Mode"=w523, "多功能校准源接口 输入"=w524) -> ()  [unwired: 8 in, 2 out]
      }
      frame "Standby" {
        w533 = u32 0 items=["Standby", "Operate"] ("Output Mode")
        n225 = Unbundle By Name(w532) -> ("个数索引"=w531:i32, "多功能校准源接口"=w534:refnum<class "多功能校准源接口.lvclass">)
        n226 = call-dynamic "Set Output Mode.vi"("Output Mode"=w533, "多功能校准源接口 输入"=w534) -> ()  [unwired: 8 in, 2 out]
        n227 = Increment(x=w531) -> (x+1=w530:i32)
        n228 = Bundle By Name(cluster=w532, "个数索引"=w530) -> (w529:T8)
      }
      frame "----------------------表-------------------" {
      }
      frame "表配置" {
        n229 = Unbundle By Name(w545) -> ("当前参数"=w552:string, "数字多用表接口"=w553:refnum<class "数字多用表接口.lvclass">, "配置数组"=w551:string[][], "个数索引"=w550:i32)
        n230 = Index Array(array=w551, index (row)=w550) -> (element=w549:string[])  [unwired: 1 in]
        n231 = call "表配置.vi"("Item"=w552, "Arguments"=w549, "数字多用表接口输入"=w553) -> ("error out"=w548:errorcluster, "delay(s)"=w542:dbl, "数字多用表接口输出"=w547:refnum<class "数字多用表接口.lvclass">)  [unwired: 6 in]
        n232 = call-dynamic "Configure.vi"("error in (no error)"=w548, "数字多用表接口 输入"=w547) -> ("数字多用表接口 输出"=w544:refnum<class "数字多用表接口.lvclass">)  [unwired: 8 in, 1 out]
        n233 = Multiply(x=1000, y=w542) -> (x*y=w541:dbl)
        n234 = Bundle By Name(cluster=w545, "Delay Time(ms)"=w541, "数字多用表接口"=w544) -> (w543:T8)
      }
      frame "Measure" {
        n235 = Unbundle By Name(w565) -> ("数字多用表接口"=w566:refnum<class "数字多用表接口.lvclass">, "MeaCount"=w562:i32)
        n236 = call-dynamic "Measure.vi"("数字多用表接口 输入"=w566) -> ("Measurement"=w564:dbl)  [unwired: 8 in, 2 out]
        n237 = Increment(x=w562) -> (x+1=w561:i32)
        n238 = Equal?(x=w561, y=3) -> (x = y?=w559:bool)
        n239 = Bundle By Name(cluster=w565, "Measurement"=w564, "MeaCount"=w561) -> (w563:T8)
        n240 = Select(t="Write MListbox" ("CMD"), s=w559, f=w557) -> (s? t:f=w556:string)
      }
      frame "---------------------MListBox------------------" {
      }
      frame "初始化表格" {
      }
      frame "Init MListbox" {
        w575 = refnum<class "MListBox.lvclass">[] []  # MLbs
        n241 = Variant To Data(type=w575, Variant=w579) -> (data=w577:refnum<class "MListBox.lvclass">[])  [unwired: 1 in, 1 out]
        n242 = Bundle By Name(cluster=w578, "MLbs"=w577) -> (w576:T8)
      }
      frame "Write MListbox" {
        n243 = Unbundle By Name(w584) -> ("MListBox"=w585:refnum<class "MListBox.lvclass">, "Measurement"=w619:dbl, "配置数组"=w617:string[][], "个数索引"=w616:i32)
        n244 = Index Array(array=w617, index (row)=w616) -> (element=w615:string[])  [unwired: 1 in]
        n245 = Index Array(array=w615, index #1=6 ("索引 (行)"), index #2=11 ("索引 (行)"), index #3=9 ("索引 (行)")) -> (element #1=w613:string, element #2=w621:string, element #3=w620:string)
        n246 = Fract/Exp String To Number(string=w621) -> (number=w618:dbl)  [unwired: 3 in, 1 out]
        n247 = Fract/Exp String To Number(string=w620) -> (number=w614:dbl)  [unwired: 3 in, 1 out]
        n248 = Divide(x=w619, y=w618) -> (x/y=w595:dbl)
        n249 = call <vilib>:"Delimited String to 1D String Array.vi"("delimiter"=",", "delimited string"=w613) -> ("string array"=w611:string[])  [unwired: 9 in]
        n250 = Number To Fractional String(number=w595, precision (6)=w614) -> (F-format string=w607:string)  [unwired: 2 in]
        n251 = Index Array(array=w611) -> (element #1=w610:string, element #2=w609:string)  [unwired: 2 in]
        n252 = Decimal String To Number(string=w610) -> (number=w586:i32)  [unwired: 2 in, 1 out]
        n253 = Decimal String To Number(string=w609) -> (number=w603:i32)  [unwired: 2 in, 1 out]
        n254 = Bundle(w586, w603) -> (w608:cluster{i32, i32})  [unwired: 1 in]
        n255 = Decrement(x=w603) -> (x-1=w606:i32)
        n256 = Increment(x=w603) -> (x+1=w602:i32)
        n257 = Bundle(w586, w606) -> (w604:cluster{i32, i32})  [unwired: 1 in]
        n258 = Bundle(w586, w602) -> (w601:cluster{i32, i32})  [unwired: 1 in]
        n259 = call <vilib>:"Get One Cell.vi"("index"=w604, "Multicolumn ListBox in"=w585) -> ("error out"=w600:errorcluster, "Cell"=w599:string, "Multicolumn ListBox out"=w605:refnum<class "MListBox.lvclass">)  [unwired: 7 in]
        n260 = Fract/Exp String To Number(string=w599) -> (number=w596:dbl)  [unwired: 3 in, 1 out]
        n261 = call <vilib>:"Get One Cell.vi"("error in (no error)"=w600, "index"=w601, "Multicolumn ListBox in"=w605) -> ("error out"=w593:errorcluster, "Cell"=w598:string, "Multicolumn ListBox out"=w594:refnum<class "MListBox.lvclass">)  [unwired: 6 in]
        n262 = Fract/Exp String To Number(string=w598) -> (number=w597:dbl)  [unwired: 3 in, 1 out]
        n263 = In Range and Coerce(upper limit=w597, x=w595, lower limit=w596) -> (In Range?=w592:bool)  [unwired: 1 out]
        n264 = Select(t=u32 16448250 ("Backcolor"), s=w592, f=u32 16711680 ("Backcolor")) -> (s? t:f=w589:u32)
        n265 = call <vilib>:"Replace Cell.vi"("Backcolor"=w589, "error in (no error)"=w593, "String"=w607, "index"=w608, "Multicolumn ListBox in"=w594) -> ("error out"=w588:errorcluster, "Multicolumn ListBox out"=w587:refnum<class "MListBox.lvclass">)  [unwired: 5 in]
        n266 = call <vilib>:"Update Index and VScrollbar.vi"("error in (no error)"=w588, "Index(Row)"=w586, "Multicolumn ListBox in"=w587) -> ()  [unwired: 7 in, 2 out]
        n267 = Bundle By Name(cluster=w584, "MeaCount"=0) -> (w582:T8)
      }
    }
    n268 = call "Queue In.vi"("error in (no error)"=w33, "Data"=w31, "Message"=w32, "Queue In"=w36) -> ("error out"=w34:errorcluster, "Queue Out"=w35:refnum<queue>)  [unwired: 6 in]
  }
  n269 = while "UI" {
    tunnel: w20 -> [w639]
    tunnel: [w636] -> w22
    tunnel: [w635] -> w21
    shift-right: [w631] -> _
    shift-left: _ -> [w630]
    tunnel: w10 -> [w628]
    stop <- w643 stop-if-true
    n270 = Unbundle By Name ("按名称解除捆绑")(w630) -> ("Queue.MNT"=w629:string)
    n271 = call "Queue Out.vi"("Monitor"=w629, "Queue In"=w639) -> ("error out"=w642:errorcluster, "Data"=w640:variant, "Message"=w641:string, "Queue Out"=w638:refnum<queue>)  [unwired: 5 in, 1 out]
    n272 = case "Case" shown="\"refresh MListbox\"" w641 {
      tunnel: w638 -> [w648 w667 w683 w688 w696 w704 w708 w712 w731 w735]
      tunnel: w642 -> [w647 w666 w682 w687 w695 w702 w709 w711 w730 w734]
      tunnel: [w648 w667 w683 w688 w696 w703 w708 w712 w731 w735] -> w637
      tunnel: [w647 w666 w682 w687 w695 w701 w709 w711 w730 w734] -> w634
      tunnel: [w646 "Clear MListbox" ("Message") _ _ _ "Quit" _ _ _ _] -> w633
      tunnel: [_ _ _ _ _ _ TRUE _ _ _] -> w643
      tunnel: [w645 _ _ _ _ _ _ _ _ _] -> w632
      tunnel: w640 -> [_ _ _ w684 w692 _ _ _ w718 _]
      tunnel: [w644 w658 w681 w685 w693 w700 w706 w710 w717 w733] -> w631
      tunnel: w630 -> [w644 _ w681 w686 w694 w700 w706 w710 w717 w733]
      tunnel: w628 -> [_ w664 _ _ _ _ _ _ _ _]
      frame Default {
        w645 = variant  # Data
        w646 = ""  # Message
        # "所有未定义的消息经过此分支被忽略"
      }
      frame "Init" {
        # "初始化，将Alin-UI中会用到的过程数据全部定义在此分支的簇中，并存储到移位寄存器中，默认加载了Alin句柄"
        n273 = disable-structure shown="Enabled" {
          disable-tunnel: "数字多用表类lvlibp" ("名称或相对路径") -> [w669 w671]
          disable-tunnel: [w668 w670] -> w661
          frame Disabled {
            n274 = call "绝对路径.vi"("相对路径"=w669) -> ("绝对路径"=w668:path)
          }
          frame Enabled {
            n275 = call <vilib>:"Application Directory.vi"() -> ("Application Directory"=w672:path)
            n276 = Build Path(base path=w672, name or relative path=w671) -> (appended path=w670:path)
          }
        }
        n277 = control-ref of="直流电压_MLb"() -> (w655:refnum<vi>)
        n278 = control-ref of="直流电流_MLb"() -> (w654:refnum<vi>)
        n279 = control-ref of="交流电压_MLb"() -> (w653:refnum<vi>)
        n280 = control-ref of="交流电流_MLb"() -> (w652:refnum<vi>)
        n281 = control-ref of="电阻_MLb"() -> (w651:refnum<vi>)
        n282 = List Folder(path=w661) -> (folder names=w663:string[])  [unwired: 3 in, 3 out]
        n283 = for {
          tunnel: w661 -> [w680]
          tunnel: w663 -> [w677] mode=indexing
          tunnel: [w677] -> w660 mode=indexing if=w676
          n284 = Build Path(base path=w680, name or relative path=w677) -> (appended path=w679:path)
          n285 = call <vilib>:"Recursive File List.vi"("pattern"="*.lvlibp", "Folder Path"=w679) -> ("Number of Files"=w678:i32)  [unwired: 5 in, 4 out]
          n286 = Greater Than 0?(x=w678) -> (x > 0?=w676:bool)
        }
        n287 = Build Array(w655, w654, w653, w652, w651) -> (w650:refnum<vi>[])
        n288 = for {
          tunnel: [w674] -> w649 mode=indexing
          tunnel: w650 -> [w673] mode=indexing
          n289 = call <vilib>:"New MListBox.vi"("MListbox Ref"=w673) -> ("Multicolumn ListBox out"=w674:refnum<class "MListBox.lvclass">)  [unwired: 9 in, 1 out]
        }
        n290 = property on="型号" class="Ring (strict)"("Strings []"=w660) -> ()  [unwired: 2 in, 2 out]
        n291 = Bundle By Name(cluster=T13 {"Queue"={"UI"=refnum, "Message"=refnum, "Data"=refnum, "Caller"=refnum, "Name"="000 Common", "Data Path"=path "", "Class Path"=path "", "SubPanel"=refnum, "Project Name"="", "MNT"="", "Title"="", "Data Source"=refnum, "Queue List"={}, "VI"=refnum, "UE"=refnum}, "MLbs"=[], "MListBox"=refnum}, "MLbs"=w649, "Queue"=w664) -> (w658:T13)
        n292 = Unbundle By Name(w658) -> ("Queue.Data"=w657:refnum<queue>)
        n293 = call "Queue In.vi"("Data"=w649, "Message"="Init MListbox", "Queue In"=w657) -> ()  [unwired: 7 in, 2 out]
      }
      frame "====System====" {
      }
      frame "Refresh Class Ref" {
        # "此消息是由Alin的Message的Refresh Class Ref发过来，主要刷新句柄中的子Alin的句柄因映射表，若不使用可以删除"
        n294 = in-place {
          in-place-border: w684 -> [w691]
          n295 = in-place-cluster #3(w686) -> ("Queue"=w690:T1)
          n296 = Variant To Data(type=w690, Variant=w691) -> (data=w689:T1)  [unwired: 1 in, 1 out]
          n297 = in-place-cluster #3("Queue"=w689) -> (w685:T13)
        }
      }
      frame "Queue Monitor" {
        # "此消息是队列监控器发来，若不使用可以删除"
        n298 = in-place {
          in-place-border: w692 -> [w699]
          n299 = in-place-cluster #4(w694) -> ("Queue.MNT"=w698:string)
          n300 = Variant To Data(type=w698, Variant=w699) -> (data=w697:string)  [unwired: 1 in, 1 out]
          n301 = in-place-cluster #4("Queue.MNT"=w697) -> (w693:T13)
        }
      }
      frame "Exit" {
        n302 = call "Queue Clear.vi"("error in (no error)"=w702, "Queue In"=w704) -> ("error out"=w701:errorcluster, "Queue Out"=w703:refnum<queue>)  [unwired: 8 in]
      }
      frame "Quit" {
      }
      frame "====User====" {
      }
      frame "refresh MListbox" {
        n303 = Variant To Data(type=T12 {"MListBox"=refnum, "Values"=[]} ("output cluster"), Variant=w718) -> (data=w715:T12)  [unwired: 1 in, 1 out]
        n304 = Unbundle By Name(w715) -> ("Values"=w713:string[][], "MListBox"=w714:refnum<class "MListBox.lvclass">)
        n305 = call <vilib>:"Clear All Rows.vi"("BackColors"=cluster{"OddRow Color":u32, "EvenRow Color":u32} {"OddRow Color"=16448250, "EvenRow Color"=16448250}, "Multicolumn ListBox in"=w714) -> ("error out"=w728:errorcluster, "Multicolumn ListBox out"=w727:refnum<class "MListBox.lvclass">)  [unwired: 8 in]
        n306 = call <vilib>:"Insert Rows.vi"("error in (no error)"=w728, "Rows"=w713, "Index"=i16 0, "Multicolumn ListBox in"=w727) -> ("error out"=w721:errorcluster, "Multicolumn ListBox out"=w720:refnum<class "MListBox.lvclass">)  [unwired: 5 in, 1 out]
        n307 = call <vilib>:"Autosize Column Width.vi"("error in (no error)"=w721, "Autosize Mode"=Autosize_Mode."All Cells", "Multicolumn ListBox in"=w720) -> ("error out"=w724:errorcluster, "Multicolumn ListBox out"=w723:refnum<class "MListBox.lvclass">)  [unwired: 7 in]
        n308 = call <vilib>:"Align Columns.vi"("Active Cell:Cell Justification"=enum16{"Left", "Center", "Right"}."Center", "error in (no error)"=w724, "Column Index"=i16 -1, "Multicolumn ListBox in"=w723) -> ()  [unwired: 6 in, 2 out]
      }
      frame "Clear MListbox" {
        n309 = Unbundle By Name(w733) -> ("MLbs"=w732:refnum<class "MListBox.lvclass">[])
        n310 = for {
          tunnel: w732 -> [w736] mode=indexing
          n311 = call <vilib>:"Clear All Rows.vi"("BackColors"=cluster{"OddRow Color":u32, "EvenRow Color":u32} {"OddRow Color"=16448250, "EvenRow Color"=16448250}, "Multicolumn ListBox in"=w736) -> ()  [unwired: 8 in, 2 out]
        }
      }
    }
    n312 = call "Queue In.vi"("error in (no error)"=w634, "Data"=w632, "Message"=w633, "Queue In"=w637) -> ("error out"=w635:errorcluster, "Queue Out"=w636:refnum<queue>)  [unwired: 6 in]
  }
  n313 = while "UE" {
    tunnel: w25 -> [w741]
    tunnel: [w739] -> w24
    tunnel: w10 -> [w738]
    stop <- w740 stop-if-true
    n314 = event "Event" shown="[4] \"测量\": Value Change" {
      selector: w741 -> [_ _ _ _ _ _ _ _ _ _ _ _ _]
      dyn-events: [_ _ _ _ _ _ _ _ _ _ _ _ _] -> w739
      timeout: _ -> [_ _ _ _ _ _ _ _ _ _ _ _ _]
      tunnel: [_ _ _ _ _ _ _ _ w780 _ _ _ _] -> w740
      tunnel: w738 -> [_ w742 w749 w752 w755 w758 w759 _ _ w787 w803 w806 w809]
      event Timeout {
        n315 = event-data() -> ()  [unwired: 1 in, 1 out]
      }
      event Key Down {
        # "所有界面上按键按下事件的处理"
        n316 = event-data() -> ("Char"=w745:i16, "VKey"=w746:T15, "Mods"=w744:cluster{"Num Pad":bool, "Menu Key":bool}, "PlatMods"=w743:T16)  [unwired: 1 in]
        n317 = call "Queue Key Down.vi"("Queue Ref Out"=w742, "C"=w745, "Platform Key"=w743, "Group Key"=w744, "V Key"=w746) -> ()  [unwired: 6 in, 1 out]
      }
      event Value Change {
        n318 = event-data() -> ()  [unwired: 1 in, 1 out]
        n319 = Unbundle By Name ("按名称解除捆绑")(w749) -> ("Data"=w748:refnum<queue>)
        n320 = call "Queue In.vi"("Message"="Connect", "Queue In"=w748) -> ()  [unwired: 8 in, 2 out]
      }
      event Value Change {
        n321 = event-data() -> ()  [unwired: 1 in, 1 out]
        n322 = Unbundle By Name ("按名称解除捆绑")(w752) -> ("Data"=w751:refnum<queue>)
        n323 = call "Queue In.vi"("Message"="Load", "Queue In"=w751) -> ()  [unwired: 8 in, 2 out]
      }
      event Value Change {
        n324 = event-data() -> ()  [unwired: 1 in, 1 out]
        n325 = Unbundle By Name ("按名称解除捆绑")(w755) -> ("Data"=w754:refnum<queue>)
        n326 = call "Queue In.vi"("Message"="判断参数", "Queue In"=w754) -> ()  [unwired: 8 in, 2 out]
      }
      event "保存": Value Change {
        n327 = event-data() -> ()  [unwired: 1 in, 1 out]
        n328 = Unbundle By Name ("按名称解除捆绑")(w758) -> ("Data"=w757:refnum<queue>)
        n329 = call "Queue In.vi"("Message"="Save", "Queue In"=w757) -> ()  [unwired: 8 in, 2 out]
      }
      event "测量参数": Value Change {
        n330 = event-data() -> ()  [unwired: 1 in, 1 out]
        n331 = Unbundle By Name ("按名称解除捆绑")(w759) -> ("Data"=w761:refnum<queue>)
        n332 = call "Queue In.vi"("Message"="测量参数", "Queue In"=w761) -> ()  [unwired: 8 in, 2 out]
      }
      event "待选参数": Shortcut Menu Selection (User) {
        n333 = event-data() -> ("CtlRef"=w763:refnum<vi>, "ItemTag"=w766:string, "Coords"=w765:T17)  [unwired: 1 in]
        n334 = invoke on="待选参数" class="LstBox (strict)" method="Point To Row"("Point"=w765) -> ("InBounds"=w764:bool, "Row"=w762:i32)  [unwired: 6 in, 5 out]
        n335 = case shown="True" w764 {
          tunnel: w766 -> [_ w769]
          tunnel: w763 -> [_ w768]
          tunnel: w762 -> [_ w767]
          frame False {
          }
          frame True {
            n336 = case shown="\"启用\"" w769 {
              tunnel: w768 -> [_ w774 w779]
              tunnel: w767 -> [_ w772 w777]
              frame "False", Default {
              }
              frame "禁用" {
                n337 = property class="LstBox (strict)"(reference=w774) -> (reference out=w771:refnum<vi>, "Disabled Items"=w773:i32[])  [unwired: 1 in, 1 out]
                n338 = Build Array (concatenate)(w773, w772) -> (w770:i32[])
                n339 = property class="LstBox (strict)"(reference=w771, "Disabled Items"=w770) -> ()  [unwired: 1 in, 2 out]
              }
              frame "启用" {
                n340 = property class="LstBox (strict)"(reference=w779) -> (reference out=w778:refnum<vi>, "Disabled Items"=w776:i32[])  [unwired: 1 in, 1 out]
                n341 = call-poly <userlib>:"Filter 1D Array__ogtk.vi"("items to filter"=w777, "array"=w776) -> ("filtered array"=w775:i32[])  [unwired: 4 in, 1 out]
                n342 = property class="LstBox (strict)"(reference=w778, "Disabled Items"=w775) -> ()  [unwired: 1 in, 2 out]
              }
            }
          }
        }
      }
      event User Event {
        # "此分支有Alin的Message线程发送过来用来退出用户事件所在的线程"
        n343 = event-data() -> ("Message"=w782:string)  [unwired: 1 in]
        n344 = Equal?(x=w782, y="Exit") -> (x = y?=w780:bool)
      }
      event Panel Close? {
        # "用户点击前面板关闭的按键"
        n345 = event-data() -> ()  [unwired: 1 in, 1 out]
        n346 = property class="App"() -> ("App.Kind"=w786:T14)  [unwired: 2 in, 2 out]
        n347 = Equal?(x=w786, y=T14."Run Time System") -> (x = y?=w785:bool)
        n348 = case shown="True" w785 {
          tunnel: [TRUE ("T button?") w801] -> w783
          frame False {
          }
          frame True {
            n349 = Two Button Dialog(message="确定要退出程序吗？" ("消息")) -> (T button?=w801:bool)  [unwired: 2 in]
          }
        }
        n350 = case shown="True" w783 {
          tunnel: w787 -> [_ w791]
          frame False {
          }
          frame True {
            n351 = Call Chain() -> (call chain=w793:string[])
            n352 = Array Size(array=w793) -> (size(s)=w792:i32)
            n353 = case shown="2, Default" w792 {
              tunnel: w791 -> [w796 w799]
              tunnel: [w795 w798] -> w790
              tunnel: ["Panel Hidden" ("Message") "Exit Prepare" ("Message")] -> w789
              frame 2, Default {
                # "当调用链大于2的时候，只隐藏前面板"
                n354 = Unbundle By Name(w796) -> ("Message"=w795:refnum<queue>)
              }
              frame 1 {
                # "只打开此Alin的时候使用默认退出"
                n355 = Unbundle By Name(w799) -> ("Message"=w798:refnum<queue>)
              }
            }
            n356 = call "Queue In.vi"("Message"=w789, "Queue In"=w790) -> ()  [unwired: 8 in, 2 out]
          }
        }
        n357 = event-data("Discard?"=TRUE ("放弃？")) -> ()  [unwired: 1 in, 1 out]
      }
      event Value Change {
        n358 = event-data() -> ()  [unwired: 1 in, 1 out]
        n359 = Unbundle By Name ("按名称解除捆绑")(w803) -> ("Data"=w805:refnum<queue>)
        n360 = call "Queue In.vi"("Message"="复位", "Queue In"=w805) -> ()  [unwired: 8 in, 2 out]
      }
      event "暂停": Value Change {
        n361 = event-data() -> ()  [unwired: 1 in, 1 out]
        n362 = Unbundle By Name ("按名称解除捆绑")(w806) -> ("Data"=w808:refnum<queue>)
        n363 = call "Queue In.vi"("Message"="暂停", "Queue In"=w808) -> ()  [unwired: 8 in, 2 out]
      }
      event Value Change {
        n364 = event-data() -> ()  [unwired: 1 in, 1 out]
        n365 = Unbundle By Name ("按名称解除捆绑")(w809) -> ("Data"=w811:refnum<queue>)
        n366 = call "Queue In.vi"("Message"="打开报告", "Queue In"=w811) -> ()  [unwired: 8 in, 2 out]
      }
    }
  }
  n367 = call "000 Driver Message.vi"("Queue In"=w10) -> ("error out"=w13:errorcluster)  [unwired: 8 in, 2 out]
  n368 = call "Queue Release.vi"("error in (no error)"=w16, "Queue In"=w17) -> ("error out"=w14:errorcluster)  [unwired: 9 in]
  n369 = Unregister For Events ("取消注册事件")(event registration refnum=w24) -> (error out=w23:errorcluster)  [unwired: 1 in]
  n370 = call "Queue Release.vi"("error in (no error)"=w21, "Queue In"=w22) -> ("error out"=w18:errorcluster)  [unwired: 9 in]
  n371 = Destroy User Event ("销毁用户事件")(user event=w12, error in=w23) -> (error out=w19:errorcluster)
  n372 = Merge Errors ("合并错误")(w19, w18, w13, w14) -> (w2:errorcluster)
  n373 = property class="App"(error in=w2) -> (error out=w3:errorcluster, "App.Kind"=w4:T14)  [unwired: 1 in, 1 out]
  n374 = case shown="\"invalid app kind\", Default" w4 {
    tunnel: w3 -> [w812 _]
    frame "invalid app kind", Default {
      n375 = invoke class="VI" method="FP.Close"(error in=w812) -> ()  [unwired: 2 in, 3 out]
    }
    frame "Development System" {
    }
  }
